vi "eodrecorder_sarah_sam - Timed (2012).vi"() -> ()   [LabVIEW 2013]
uses:
  Dependencies/eodrecorderstates.ctl
  <vilib>/Utility/error.llb/DialogType.ctl
  <vilib>/_DAQmxBase/Internals/DAQmxBase Create Channel (AI-Voltage-Basic).vi
  <vilib>/_DAQmxBase/Internals/DAQmxBase Timing (Sample Clock).vi
  <vilib>/_DAQmxBase/Internals/DAQmxBase Read (Analog 2D DBL NChan NSamp).vi
panel:
  out "String":string
  in  "Length":dbl=0.05
  in  "Device in":tag="Dev1"
  out "Threshold":sgl
  out "?":string="10 E"
  in  "Multiplier":sgl min=-2 max=0
  in  "Modify\nThreshold":dbl(slide) min=0.0 max=9.0 step=1.0 scale=0.0..9.0 scale format="%#_1g"
  in  "?":bool
  out "Number\nof Samples":sgl=10000.0
  in  "Sample Rate":dbl=10000.0
  in  "Channel":tag="Dev1/ai0"
  out "Tab Control":enum32{"Live Data", "Edit Data", "View Data"}(tab)
  in  "Tab Control 2":enum32{"Enter Data", "View Data"}(tab)
  out "Waveforms\nCollected":dbl
  in  "Path":path
  out "Time":string
  out "Date":string
  in  "Specimen No.":string
  in  "Locality Code":string
  in  "Gain":dbl(knob)=10000.0 step=1.0 scale=1.0..50000.0 scale format="%#_6e"
  in  "Coupling":bool
  in  "Recording Temp °C":string
  in  "Comments":string
  in  "Species":string
  in  "StartOver":bool
  in  "Save&Continue":bool
  in  "Save&Finish":bool
  in  "Discard&Continue":bool
  in  "Polarity 2":bool
  in  "Timed":bool
  out "Number of \nWaveforms":dbl caption="Number of Waveforms" format="%#g"
  in  "Wave Number":u16(slide) scale=0.0..1.0
  in  "Polarity":bool
  out "EodText":string[](array[string])
  out "Polarity":i32[](array[numeric])
  out "Npts":i32[](array[numeric])
  out "Srate":i32[](array[numeric])
  out "ADRange":dbl[](array[numeric])
  in  "WaveNumber":i32(slide)=1 min=0 step=1 scale=1.0..3.0 scale format="%#.0f"
  out "Waveform Graph":dbl[][](graph)
  in  "LiveDataMode":bool
  in  "Capture":bool
  in  "Stop":bool
  in  "Open Data":bool
  # "EOD Recorder v. 1.0"
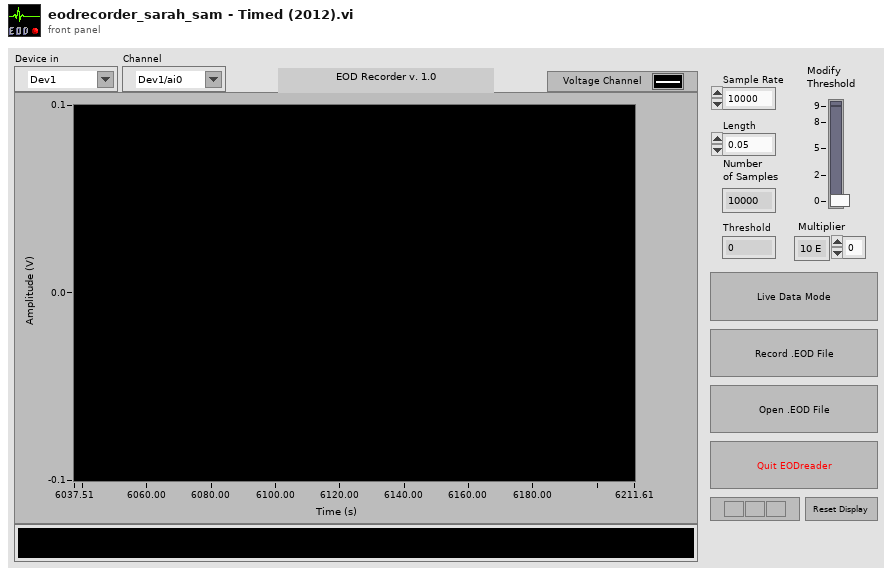
[diagram p1: front panel]
types:
  T1 = cluster{"data":dbl[][], "task ":refnum<k21>, "error ":errorcluster, "Min":dbl, "Max":dbl, "LastGrabbedSrate":dbl, "WaveformData":cluster{"Nchar":i32[], "EodText":string[], "Nbits":i32[], "Nbytes":i32[], "userdata":dbl[][], "Polarity":i32[], "Srate":i32[], "ADRange":dbl[], "Npts":i32[], "Wave":dbl[][]}, "NumberofWavesLoaded":i32, "DescribeWave":cluster{"Specimen 2":string, "Location 2":string, "Species 2":string, "Temp 2":string, "Comments 2":string, "Gain 2":dbl, "Coupling 2":bool, "Date 2":string, "Time 2":string, "Srate 2":dbl, "Polarity 2":bool, "npts":i32}[], "lastgrabbedsamples":i32}
  T2 = typedef "eodrecorderstates.ctl" = enum16{"stop", "initialize", "live data", "capture data", "analyze data", "open data", "display opened data", "write to file"}
  T3 = enum16{"Rising Edge", "Falling Edge", "Above Level", "Below Level", "When Inside Window", "When Outside Window"}
  T4 = enum16{"open", "replace", "create", "open or create", "replace or create", "replace or create with confirmation"}
  T5 = cluster{"Specimen 2":string, "Location 2":string, "Species 2":string, "Temp 2":string, "Comments 2":string, "Gain":dbl, "Coupling":bool, "Date 2":string, "Time 2":string, "Srate":dbl, "Polarity":bool, "npts":i32}
  T6 = typedef "DialogType.ctl" = u16
  T7 = cluster{"Nchar":i32[], "EodText":string[], "Nbits":i32[], "Nbytes":i32[], "userdata":dbl[][], "Polarity":i32[], "Srate":i32[], "ADRange":dbl[], "Npts":i32[], "Wave":dbl[][]}
  T8 = typedef "eventvkey.ctl" = enum16{"ASCII", "Enter", "Return", "Shift", "Ctrl", "Alt", "Cmd", "Opt", "Caps", "NumLock", "Clear", "Break", "Up", "Down", "Left", "Right", "Insert", "Delete", "Home", "End", "PageUp", "PageDown", "Escape", "Help", "Pause", "ScrollLock", "F1", "F2", "F3", "F4", "F5", "F6", "F7", "F8", "F9", "F10", "F11", "F12", "F13", "F14", "F15", "F16", "F17", "F18", "F19", "F20", "F21", "F22", "F23", "F24", "Play", "VolumeUp", "VolumeDown", "Mute", "Two Byte Char"}
  T9 = cluster{"Specimen 2":string, "Location 2":string, "Species 2":string, "Temp 2":string, "Comments 2":string, "Gain 2":dbl, "Coupling 2":bool, "Date 2":string, "Time 2":string, "Srate 2":dbl, "Polarity 2":bool, "npts":i32}[]
  T10 = cluster{"Specimen 2":string, "Location 2":string, "Species 2":string, "Temp 2":string, "Comments 2":string, "Gain 2":dbl, "Coupling 2":bool, "Date 2":string, "Time 2":string, "Srate 2":dbl, "Polarity 2":bool, "npts":i32}
  T11 = cluster{"[0]":bool, "[1]":bool, "[2]":bool, "[3]":bool, "[4]":bool, "[5]":bool, "[6]":bool, "[7]":bool, "[8]":bool}
  T12 = cluster{"Time 2":string, "Date 2":string, "Specimen 2":string, "Location 2":string, "Species 2":string, "Temp 2":string, "Gain 2":dbl, "Coupling 2":bool, "Comments 2":string}
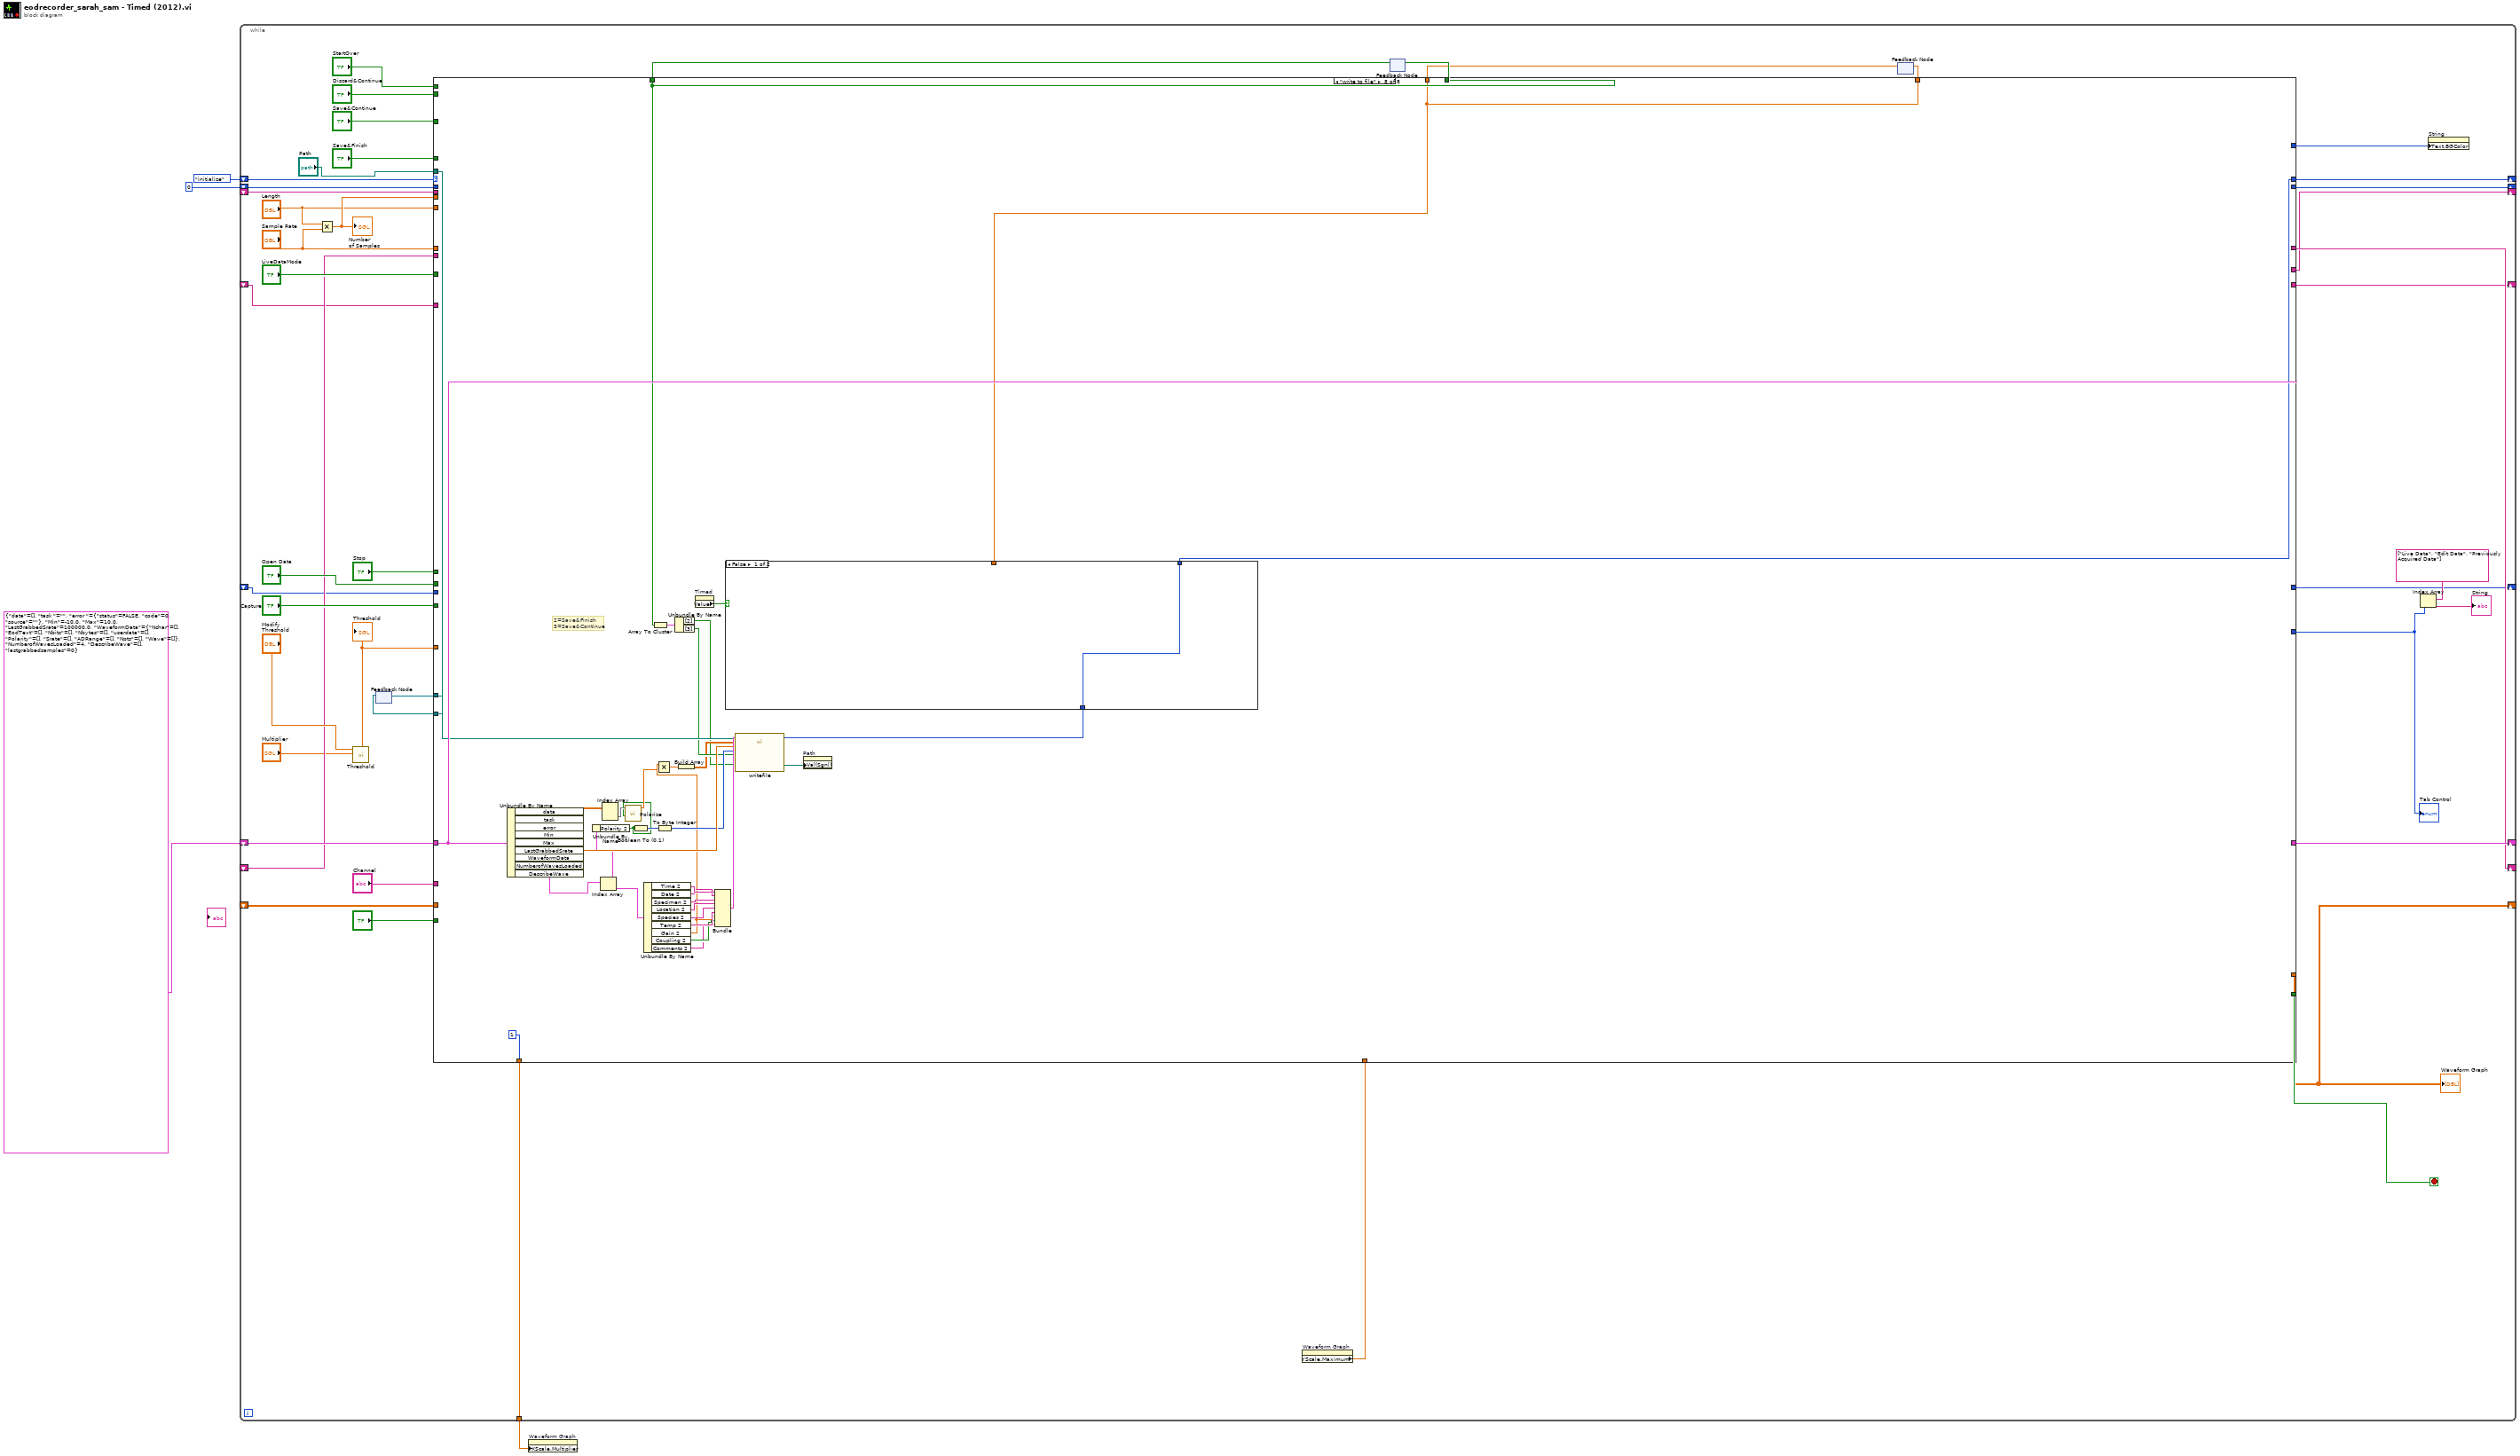
[diagram p0: block diagram]
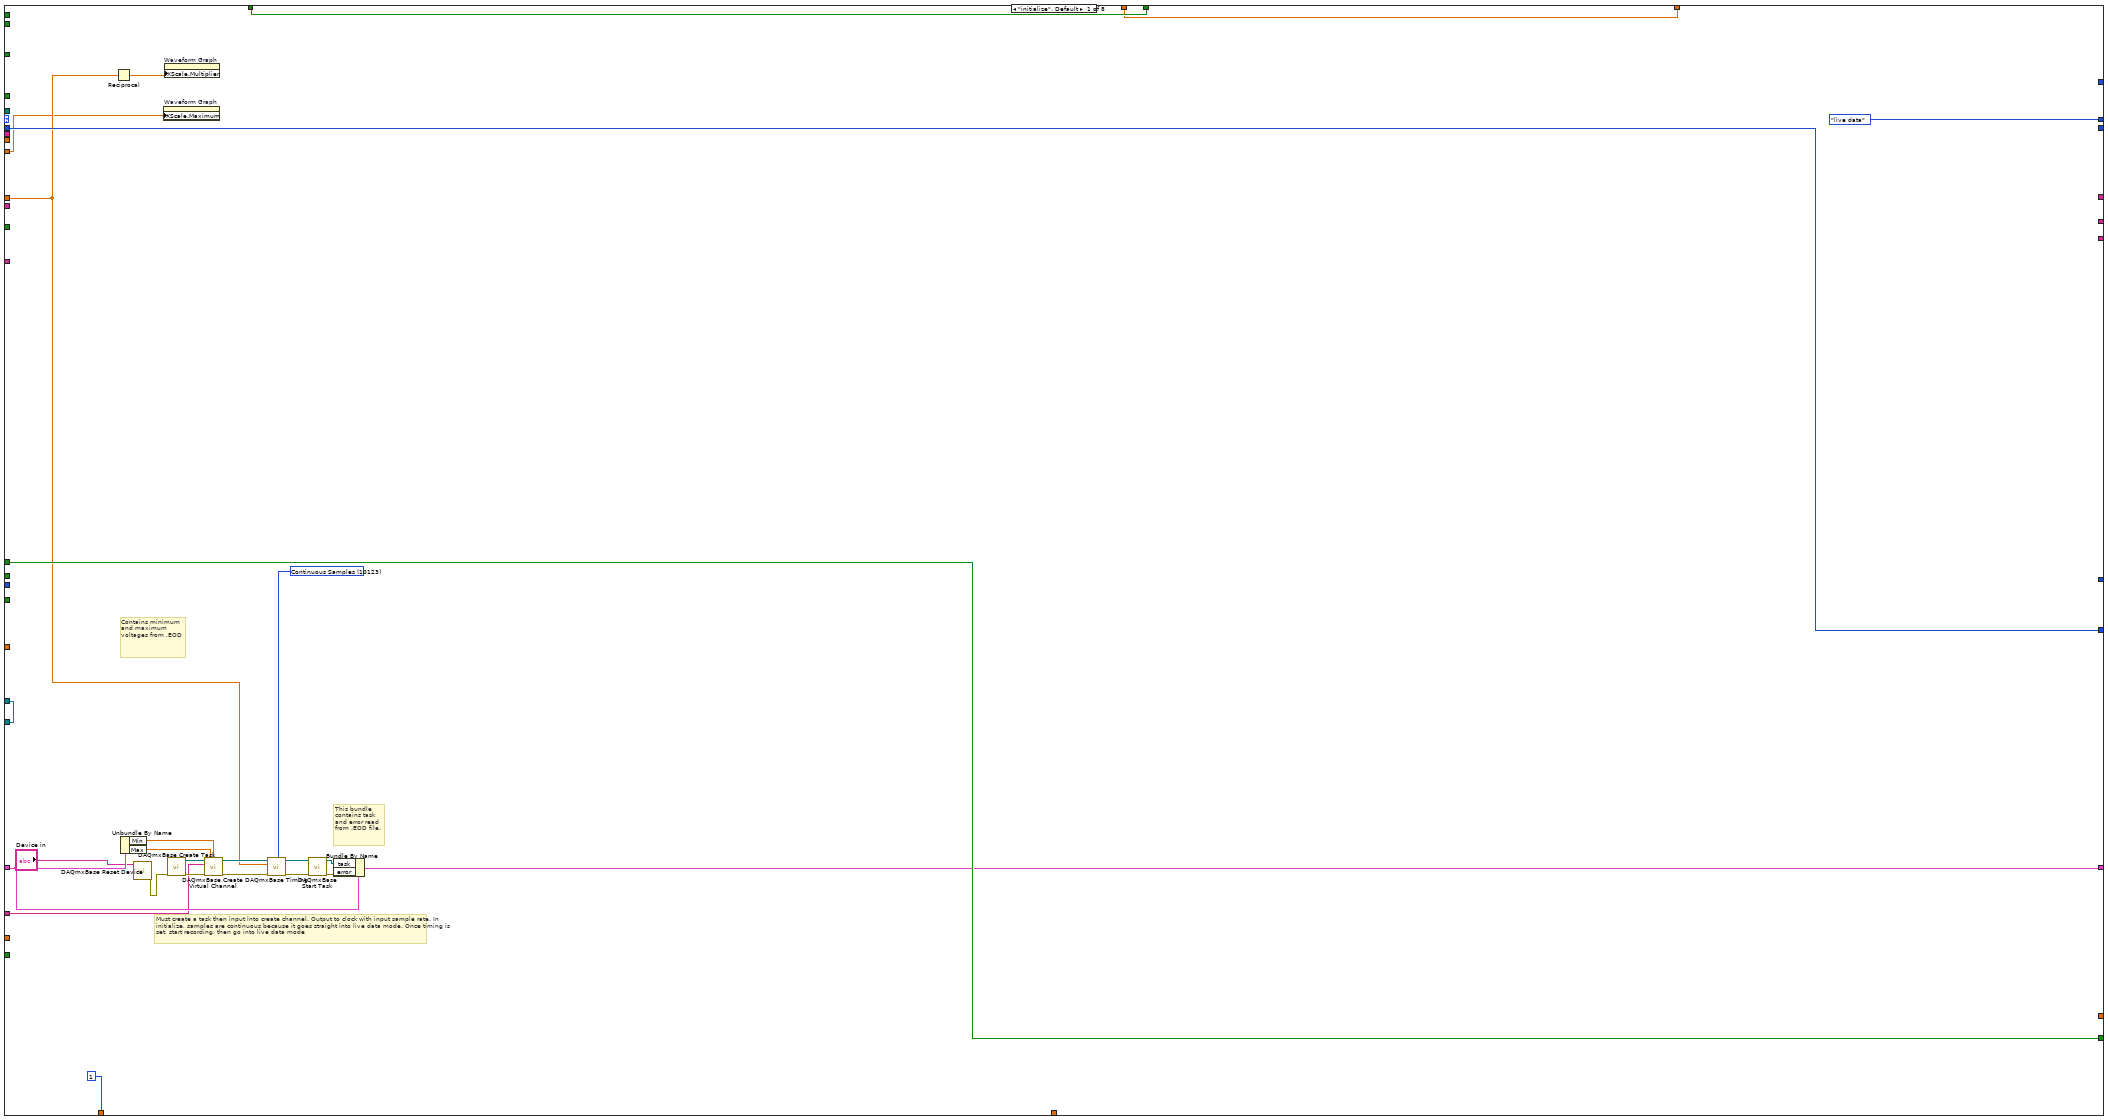
[diagram p2: hidden frame]
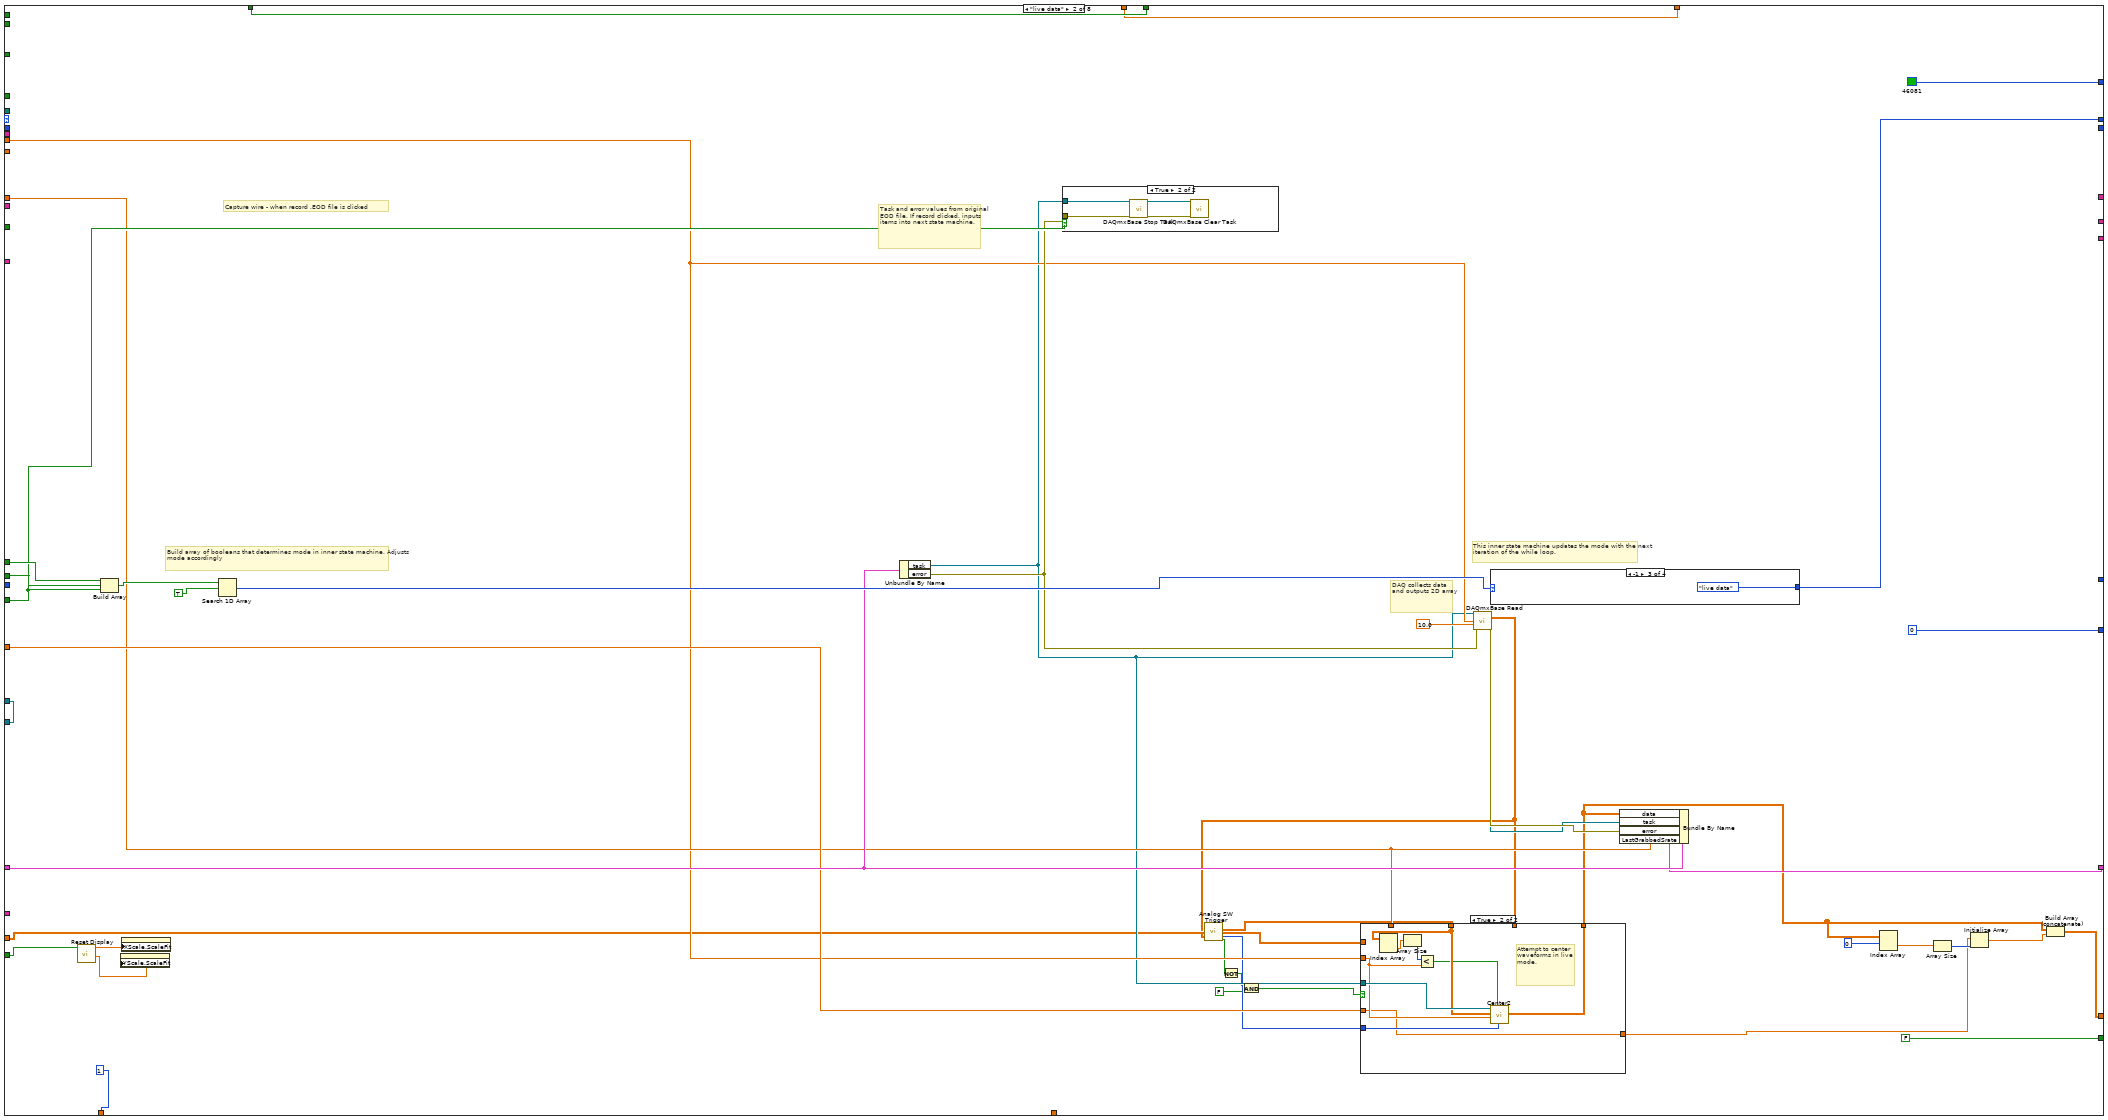
[diagram p3: hidden frame]
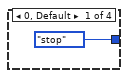
[diagram p6: hidden frame]
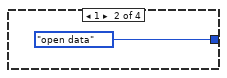
[diagram p7: hidden frame]
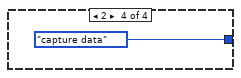
[diagram p8: hidden frame]
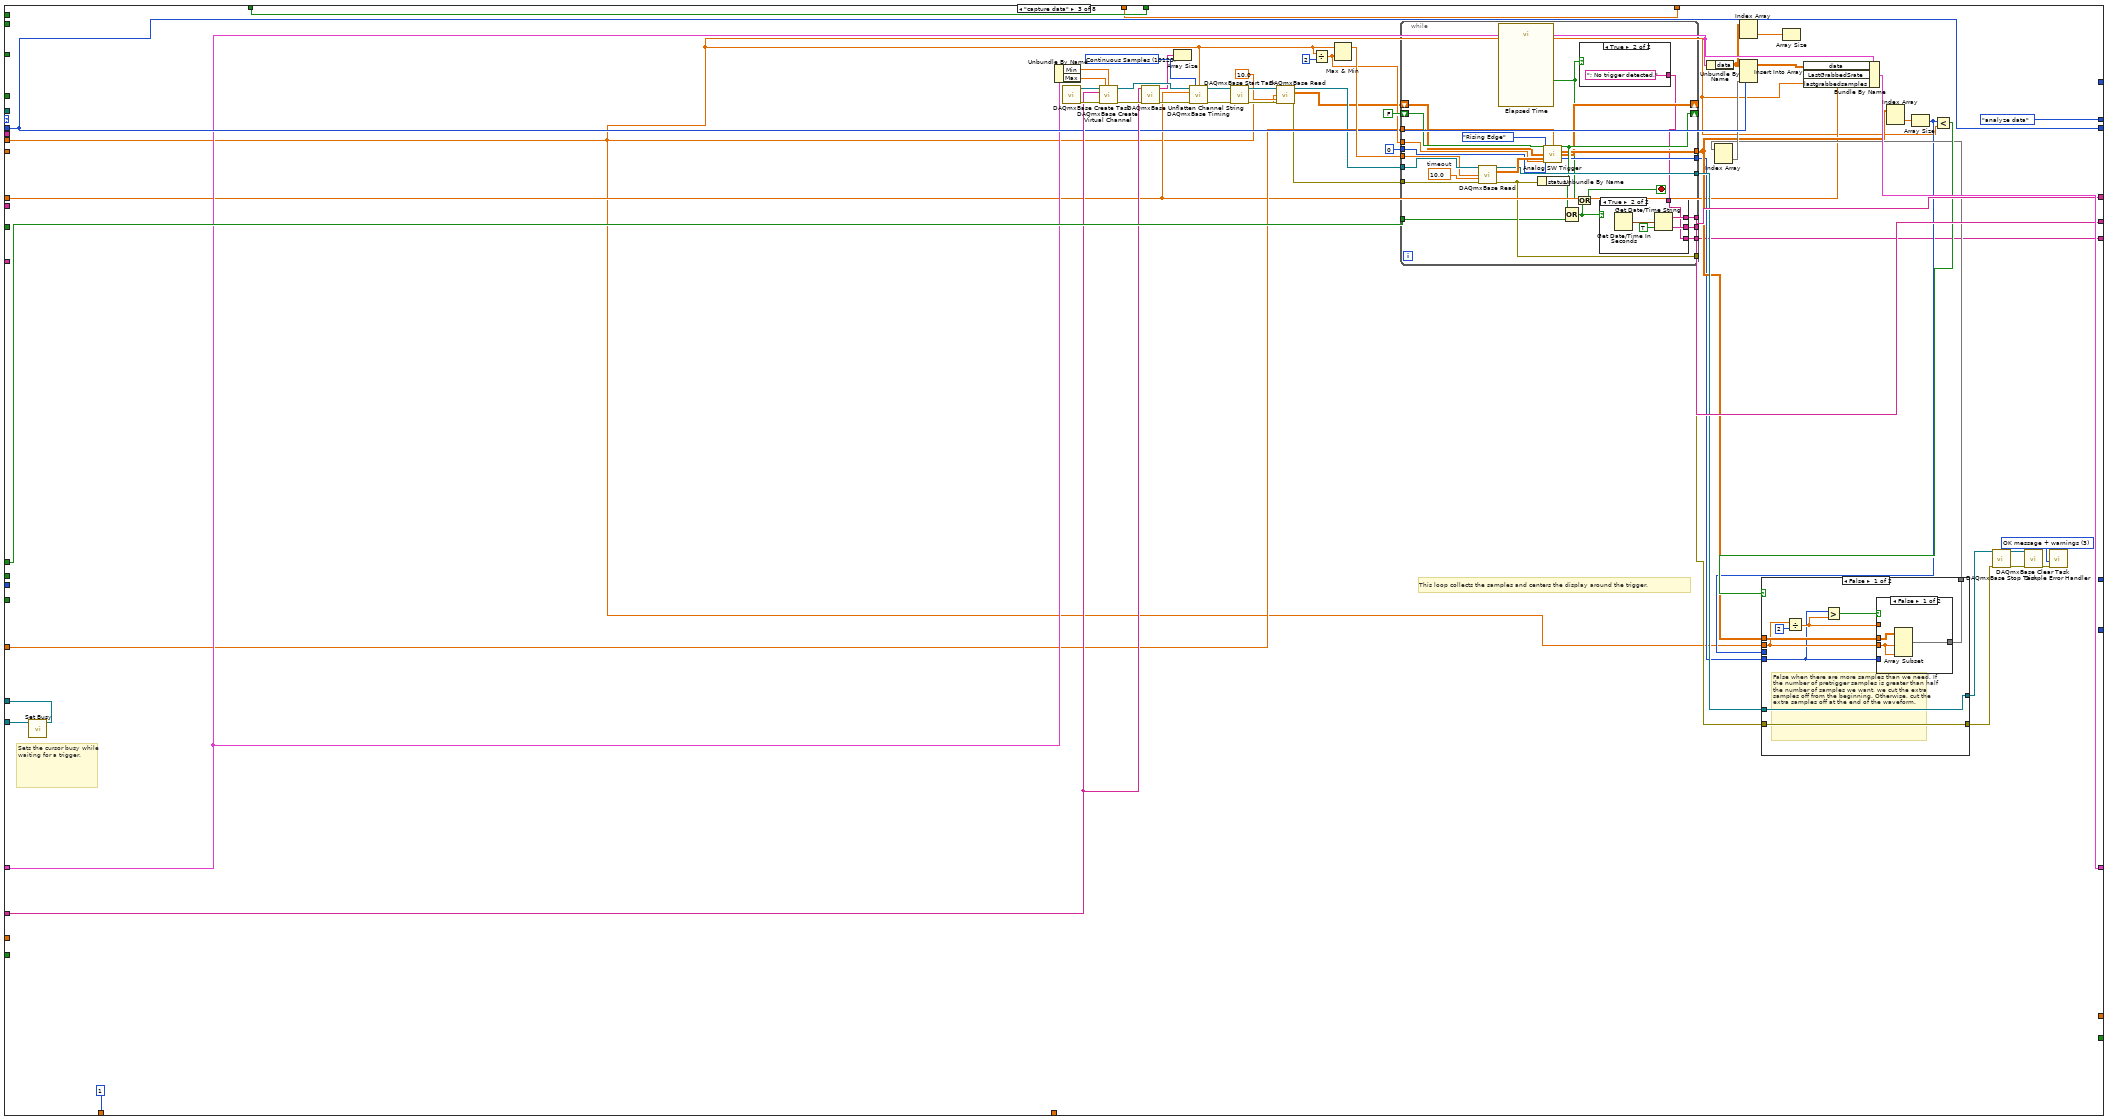
[diagram p9: hidden frame]
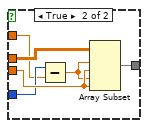
[diagram p10: hidden frame]
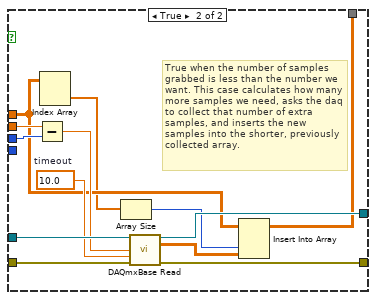
[diagram p11: hidden frame]
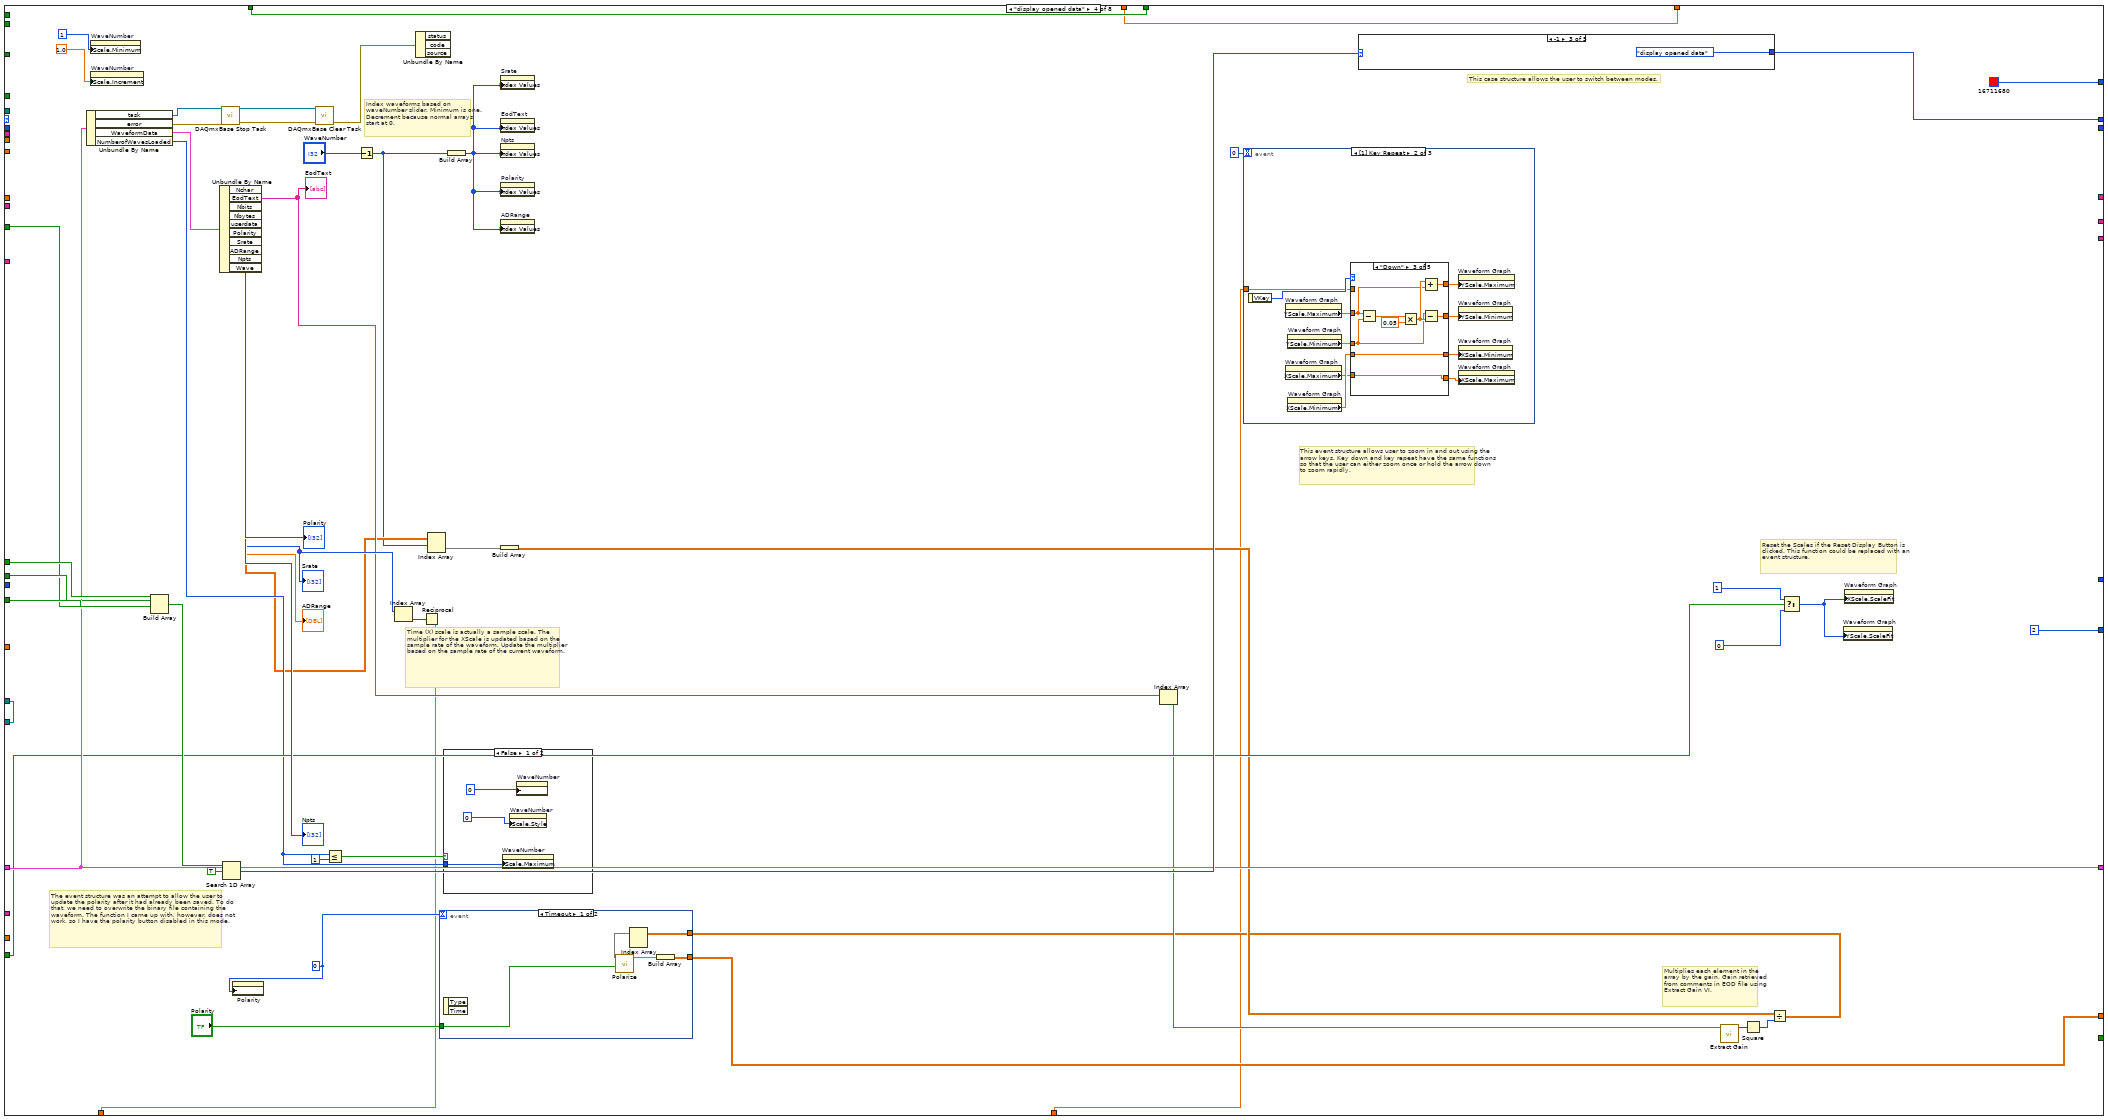
[diagram p14: hidden frame]
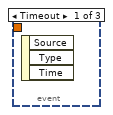
[diagram p15: hidden frame]
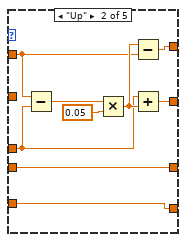
[diagram p17: hidden frame]
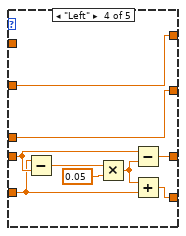
[diagram p18: hidden frame]
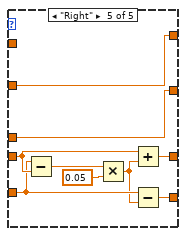
[diagram p19: hidden frame]
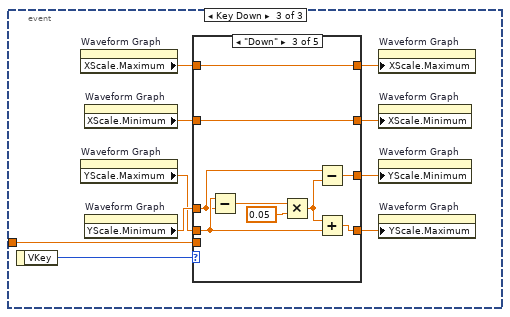
[diagram p20: hidden frame]
diagram:
  n1 = while {
    shift-right: [w49] -> _
    shift-left: eodrecorderstates."initialize" ("Enum") -> [w44]
    shift-right: [w37] -> _
    shift-left: T1 {"data"=[], "task "="", "error "={"status"=FALSE, "code"=0, "source"=""}, "Min"=-10.0, "Max"=10.0, "LastGrabbedSrate"=100000.0, "WaveformData"={"Nchar"=[], "EodText"=[], "Nbits"=[], "Nbytes"=[], "userdata"=[], "Polarity"=[], "Srate"=[], "ADRange"=[], "Npts"=[], "Wave"=[]}, "NumberofWavesLoaded"=4, "DescribeWave"=[], "lastgrabbedsamples"=0} -> [w47]
    shift-right: [w38] -> _
    shift-left: u16 0 -> [w39]
    shift-right: [w35] -> _
    shift-left: _ -> [w26]
    shift-right: [w34] -> _
    shift-left: _ -> [w33]
    shift-right: [w24] -> _
    shift-left: _ -> [w22]
    shift-right: [w12] -> _
    shift-left: _ -> [w11]
    shift-right: [w7] -> _
    shift-left: _ -> [w6]
    tunnel: [w5] -> w1
    stop <- w50 stop-if-true
    n2 = Multiply(x="Length", y="Sample Rate") -> (x*y=w29:dbl)
    "Number\nof Samples" <- w29
    n3 = call "Threshold.vi"("Multiplier"="Multiplier", "Slide"="Modify\nThreshold") -> ("New Threshold"=w27:dbl)  [unwired: 9 in]
    "Threshold" <- w27
    n4 = feedback #1() -> (w15:refnum<k1>)  [unwired: 1 in]
    n5 = property on="Waveform Graph" class="WFGraph (strict)"() -> ("YScale.Maximum"=w8:dbl)  [unwired: 2 in, 2 out]
    n6 = feedback #2() -> (w13:bool[])  [unwired: 1 in]
    n7 = feedback #3() -> (w9:dbl)  [unwired: 1 in]
    n8 = case shown="\"write to file\"" w44 {
      tunnel: [w75 FALSE _ _ _ TRUE w536 _] -> w50
      tunnel: [eodrecorderstates."live data" ("Enum") w118 eodrecorderstates."analyze data" ("Enum") w309 w442 _ w494 w718] -> w49
      tunnel: "Stop" -> [w75 w117 w178 w303 _ _ w536 _]
      tunnel: w47 -> [w63 w113 w169 w286 w440 _ w535 w748]
      tunnel: w29 -> [_ w96 w143 _ _ _ _ _]
      tunnel: "Sample Rate" -> [w56 w99 w152 _ _ _ _ _]
      tunnel: "Open Data" -> [_ w111 _ w305 _ _ _ _]
      tunnel: "Capture" -> [_ w110 _ w306 _ _ _ _]
      tunnel: "LiveDataMode" -> [_ _ _ w302 _ _ _ _]
      tunnel: w27 -> [_ w100 w168 _ _ _ _ _]
      tunnel: [w62 0 _ 2 _ _ 1 _] -> w41
      tunnel: [_ u32 46081 _ u32 16711680 _ _ u32 16773632 _] -> w40
      tunnel: w39 -> [w62 _ w170 _ _ _ w505 _]
      tunnel: [_ _ w170 _ _ _ w503 _] -> w38
      tunnel: [w60 w106 w173 w286 w439 _ w534 w748] -> w37
      tunnel: "Channel" -> [w61 _ w174 _ _ _ _ _]
      tunnel: [_ _ w172 _ _ _ w524 _] -> w35
      tunnel: [_ _ w171 _ _ _ w523 _] -> w34
      tunnel: w26 -> [_ _ _ _ _ _ w524 _]
      tunnel: w33 -> [_ _ _ _ _ _ w523 _]
      tunnel: [_ w80 _ w266 _ _ w513 _] -> w24
      tunnel: "?" -> [_ w103 _ w283 _ _ w511 _]
      tunnel: "Length" -> [w55 _ _ _ _ _ _ _]
      tunnel: w22 -> [_ w92 _ _ _ _ _ _]
      tunnel: "StartOver" -> [_ _ _ _ _ _ _ _]
      tunnel: "Save&Continue" -> [_ _ _ _ _ _ _ _]
      tunnel: "Save&Finish" -> [_ _ _ _ _ _ _ _]
      tunnel: "Discard&Continue" -> [_ _ _ _ _ _ _ _]
      tunnel: "Path" -> [_ _ _ _ _ _ w497 w731]
      tunnel: [1 1 1 w262 1 1 1 1] -> w5
      tunnel: [w53 w97 w149 w277 w436 w484 w509 w728] -> w16
      tunnel: w15 -> [w53 w97 w150 w277 w436 w484 w509 w728]
      tunnel: [w52 w78 w148 w274 w435 w483 w498 w725] -> w14
      tunnel: w13 -> [w52 w78 w148 w274 w435 w483 _ w725]
      tunnel: [_ _ _ _ w433 _ _ _] -> w12
      tunnel: w11 -> [_ _ _ _ _ _ _ _]
      tunnel: [w51 w77 w147 w263 w432 w482 w496 w716] -> w10
      tunnel: w9 -> [w51 w77 w147 w263 w432 w482 w490 w716]
      tunnel: w8 -> [_ _ _ w261 _ _ w489 _]
      tunnel: [_ _ w139 _ _ _ _ _] -> w7
      tunnel: w6 -> [_ _ _ _ _ _ w487 _]
      frame "initialize", Default {
        w70 = 10123 items=["Finite Samples"=10178, "Continuous Samples"=10123] ("sample mode")
        # "Must create a task then input into create channel. Output to clock with input sample rate. In initialize, samples are continuous because it goes straight into live data mode. Once timing is set, start recording, then go into live data mode"
        # "Contains minimum and maximum voltages from .EOD"
        # "This bundle contains task and error read from .EOD file."
        n9 = Reciprocal(x=w56) -> (1/x=w57:dbl)
        n10 = Unbundle By Name(w63) -> ("Min"=w67:dbl, "Max"=w66:dbl)
        n11 = call <vilib>:"DAQmxBase Reset Device.vi"("device in"="Device in") -> ("error out"=w58:errorcluster)  [unwired: 14 in]
        n12 = property on="Waveform Graph" class="WFGraph (strict)"("XScale.Maximum"=w55) -> ()  [unwired: 2 in, 2 out]
        n13 = property on="Waveform Graph" class="WFGraph (strict)"("XScale.Multiplier"=w57) -> ()  [unwired: 2 in, 2 out]
        n14 = call <vilib>:"DAQmxBase Create Task.vi"("error in"=w58) -> ("task out"=w73:refnum<k21>, "error out"=w74:errorcluster)  [unwired: 4 in, 9 out]
        n15 = call-poly <vilib>:"DAQmxBase Create Virtual Channel.vi"("task in"=w73, "maximum value"=w66, "minimum value"=w67, "physical channels"=w61, "error in"=w74) -> ("task out"=w71:refnum<k21>, "error out"=w72:errorcluster)  [unwired: 4 in, 5 out]
        n16 = call-poly <vilib>:"DAQmxBase Timing.vi"("task/channels in"=w71, "sample mode"=w70, "rate"=w56, "error in"=w72) -> ("task out"=w65:refnum<k21>, "error out"=w64:errorcluster)  [unwired: 3 in, 7 out]
        n17 = call <vilib>:"DAQmxBase Start Task.vi"("task/channels in"=w65, "error in"=w64) -> ("task out"=w69:refnum<k21>, "error out"=w68:errorcluster)  [unwired: 12 out]
        n18 = Bundle By Name(cluster=w63, "task"=w69, "error"=w68) -> (w60:T1)
      }
      frame "live data" {
        # "This inner state machine updates the mode with the next iteration of the while loop."
        # "DAQ collects data and outputs 2D array"
        # "Task and error values from original EOD file. If record clicked, inputs items into next state machine."
        # "Capture wire - when record .EOD file is clicked"
        # "Build array of booleans that determines mode in inner state machine. Adjusts mode accordingly"
        n19 = call "Reset Display.vi"("Reset Button"=w103) -> ("YScale Fit"=w101:dbl, "XScale Fit"=w102:dbl)  [unwired: 9 in]
        n20 = Build Array(w117, w111, w110) -> (w116:bool[])
        n21 = property class="WFGraph (strict)"("YScale.ScaleFit"=w101) -> ()  [unwired: 2 in, 2 out]
        n22 = property class="WFGraph (strict)"("XScale.ScaleFit"=w102) -> ()  [unwired: 2 in, 2 out]
        n23 = Search 1D Array(1D array=w116, element=TRUE) -> (index of element=w114:i32)  [unwired: 1 in]
        n24 = Unbundle By Name(w113) -> ("task"=w95:refnum<k21>, "error"=w109:errorcluster)
        n25 = case shown="True" w110 {
          tunnel: w95 -> [_ w134]
          tunnel: w109 -> [_ w133]
          frame False {
          }
          frame True {
            n26 = call <vilib>:"DAQmxBase Stop Task.vi"("task/channels in"=w134, "error in"=w133) -> ("task out"=w132:refnum<k21>, "error out"=w131:errorcluster)  [unwired: 12 in]
            n27 = call <vilib>:"DAQmxBase Clear Task.vi"("task in"=w132, "error in"=w131) -> ()  [unwired: 13 in, 1 out]
          }
        }
        n28 = call-poly <vilib>:"DAQmxBase Read.vi"("task/channels in"=w95, "number of samples per channel"=w96, "timeout"=10.0, "error in"=w109) -> ("task out"=w105:refnum<k21>, "data"=w90:dbl[][], "error out"=w112:errorcluster)  [unwired: 9 out]
        n29 = call "Analog SW Trigger.vi"("Initialized Data Array"=w92, "Input Raw Data"=w90) -> ("Output Data (Scaled)"=w93:dbl[][], "Raw Data Out"=w91:dbl[][], "# Pretrigger Samples"=w94:i32, "Pre-Trigger Error"=w89:bool)  [unwired: 9 in, 1 out]
        n30 = Not(x=w89) -> (.not. x?=w88:bool)
        n31 = And(x=w88, y=FALSE) -> (x .and. y?=w87:bool)
        n32 = case shown="True" w87 {
          tunnel: w100 -> [w120 w122]
          tunnel: w93 -> [_ w127]
          tunnel: w99 -> [_ _]
          tunnel: [w121 w130] -> w81
          tunnel: w96 -> [_ w124]
          tunnel: w95 -> [_ w129]
          tunnel: w94 -> [_ w128]
          tunnel: w91 -> [_ _]
          tunnel: w90 -> [w121 _]
          tunnel: [w120 w122] -> w79
          frame False {
          }
          frame True {
            # "Attempt to center waveforms in live mode."
            n33 = Index Array(array=w127) -> (element=w126:dbl[])  [unwired: 2 in]
            n34 = Array Size(array=w126) -> (size(s)=w125:i32)
            n35 = Less?(x=w125, y=w124) -> (x < y?=w123:bool)
            n36 = call "Center2.vi"("Pretrigger Samples?"=w128, "Not enough Data?"=w123, "Num Samples"=w124, "Data In"=w127, "DAQmx Task In"=w129) -> ("Data Out"=w130:dbl[][])  [unwired: 4 in, 2 out]
          }
        }
        n37 = case shown="-1" w114 {
          tunnel: [eodrecorderstates."stop" ("Enum") eodrecorderstates."open data" ("Enum") eodrecorderstates."live data" ("Enum") eodrecorderstates."capture data" ("Enum")] -> w118
          frame 0, Default {
          }
          frame 1 {
          }
          frame -1 {
          }
          frame 2 {
          }
        }
        n38 = Bundle By Name(cluster=w113, "data"=w81, "task"=w105, "error"=w112, "LastGrabbedSrate"=w99) -> (w106:T1)
        n39 = Index Array(array=w81, index (row)=0) -> (element=w83:dbl[])  [unwired: 1 in]
        n40 = Array Size(array=w83) -> (size(s)=w84:i32)
        n41 = Initialize Array(w79, w84) -> (w82:dbl[])
        n42 = Build Array (concatenate)(w81, w82) -> (w80:dbl[][])
      }
      frame "capture data" {
        w166 = T6 3 items=["no dialog", "OK message", "continue or stop message", "OK message + warnings", "continue/stop + warnings"] ("type of dialog (OK msg:1)")
        w195 = 10123 items=["Finite Samples"=10178, "Continuous Samples"=10123] ("sample mode")
        # "Sets the cursor busy while waiting for a trigger."
        # "This loop collects the samples and centers the display around the trigger."
        n43 = call <vilib>:"Set Busy.vi"("cursor ID"=w150) -> ("previous cursor ID"=w149:refnum<k1>)  [unwired: 9 in, 1 out]
        n44 = Unbundle By Name(w169) -> ("Min"=w192:dbl, "Max"=w191:dbl)
        n45 = call <vilib>:"DAQmxBase Create Task.vi"() -> ("task out"=w194:refnum<k21>, "error out"=w193:errorcluster)  [unwired: 14 in]
        n46 = call-poly <vilib>:"DAQmxBase Create Virtual Channel.vi"("task in"=w194, "maximum value"=w191, "minimum value"=w192, "physical channels"=w174, "error in"=w193) -> ("task out"=w190:refnum<k21>, "error out"=w187:errorcluster)  [unwired: 9 in]
        n47 = call "DAQmxBase Unflatten Channel String.vi"("names in"=w174, "error in"=w187) -> ("names out"=w185:string[], "error out"=w186:errorcluster)  [unwired: 12 in]
        n48 = Array Size(array=w185) -> ()  [unwired: 1 out]
        n49 = call-poly <vilib>:"DAQmxBase Timing.vi"("task/channels in"=w190, "sample mode"=w195, "samples per channel"=w143, "rate"=w152, "error in"=w186) -> ("task out"=w189:refnum<k21>, "error out"=w188:errorcluster)  [unwired: 2 in, 7 out]
        n50 = call <vilib>:"DAQmxBase Start Task.vi"("task/channels in"=w189, "error in"=w188) -> ("task out"=w146:refnum<k21>, "error out"=w145:errorcluster)  [unwired: 12 out]
        n51 = call-poly <vilib>:"DAQmxBase Read.vi"("task/channels in"=w146, "number of samples per channel"=w143, "timeout"=10.0, "error in"=w145) -> ("task out"=w142:refnum<k21>, "data"=w140:dbl[][], "error out"=w141:errorcluster)  [unwired: 9 in]
        n52 = Divide(x=w143, y=2) -> (x/y=w176:dbl)
        n53 = Max & Min(x=w143, y=w176) -> (max(x,y)=w182:dbl)  [unwired: 1 out]
        n54 = while {
          tunnel: [w246] -> w158
          shift-right: [w245] -> _
          shift-left: FALSE ("Trigger Out") -> [w251]
          shift-right: [w232] -> _
          shift-left: w140 -> [w247]
          tunnel: w141 -> [w244]
          tunnel: w142 -> [w243]
          tunnel: w176 -> [w242]
          tunnel: 0 ("Channel Index") -> [w241]
          tunnel: w182 -> [w240]
          tunnel: [w239] -> w155
          tunnel: [w238] -> w160
          tunnel: w178 -> [w237]
          tunnel: w168 -> [w236]
          tunnel: [w234] -> w172
          tunnel: [w233] -> w171
          tunnel: [w231] -> w153
          tunnel: [w229] -> w139
          stop <- w230 stop-if-true
          w252 = 10.0  # timeout
          n55 = call-poly <vilib>:"DAQmxBase Read.vi"("task/channels in"=w243, "number of samples per channel"=w240, "timeout"=w252, "error in"=w244) -> ("task out"=w246:refnum<k21>, "data"=w248:dbl[][], "error out"=w238:errorcluster)  [unwired: 9 in]
          n56 = call "Elapsed Time"() -> ("Time has Elapsed"=w228:bool)  [unwired: 12 in, 7 out]
          n57 = Unbundle By Name(w238) -> ("status"=w250:bool)
          n58 = call "Analog SW Trigger.vi"("Triggered?"=w251, "Condition"=T3."Rising Edge", "Level"=w236, "Initialized Data Array"=w247, "Input Raw Data"=w248, "Pretrigger Samples"=w242, "Index of Condition Channel"=w241) -> ("Trigger Out"=w245:bool, "Output Data (Scaled)"=w239:dbl[][], "Raw Data Out"=w232:dbl[][], "# Pretrigger Samples"=w231:i32)  [unwired: 4 in, 1 out]
          n59 = Compound Arithmetic op=OR(w245, w250, w237) -> (w235:bool)
          n60 = Or(x=w228, y=w235) -> (x .or. y?=w230:bool)
          n61 = case shown="True" w228 {
            tunnel: [_ "; No trigger detected."] -> w227
            frame False {
            }
            frame True {
            }
          }
          n62 = case shown="True" w235 {
            tunnel: [_ w256] -> w234
            tunnel: [_ w255] -> w233
            tunnel: [_ w254] -> w229
            tunnel: w227 -> [_ w254]
            frame False {
            }
            frame True {
              n63 = Get Date/Time In Seconds() -> (seconds since 1Jan1904=w258:timestamp)
              n64 = Get Date/Time String(seconds (now)=w258, want seconds? (F)=TRUE) -> (date string=w256:string, time string=w255:string)  [unwired: 1 in]
            }
          }
        }
        n65 = Unbundle By Name(w169) -> ("data"=w162:dbl[][])
        n66 = Index Array(array=w162) -> (element=w161:dbl[])  [unwired: 2 in]
        n67 = Array Size(array=w161) -> ()  [unwired: 1 out]
        n68 = Index Array(array=w155) -> (element=w163:dbl[])  [unwired: 2 in]
        n69 = Array Size(array=w163) -> (size(s)=w151:i32)
        n70 = Less?(x=w151, y=w143) -> (x < y?=w156:bool)
        n71 = case shown="False" w156 {
          tunnel: w160 -> [w203 w226]
          tunnel: [w203 w225] -> w159
          tunnel: w158 -> [w204 w224]
          tunnel: [w204 w223] -> w157
          tunnel: w143 -> [w198 w219]
          tunnel: w155 -> [w202 w215]
          tunnel: [w201 w218] -> w154
          tunnel: w151 -> [_ w220]
          tunnel: w153 -> [w196 _]
          frame False {
            # "False when there are more samples than we need. If the number of pretrigger samples is greater than half the number of samples we want, we cut the extra samples off from the beginning. Otherwise, cut the extra samples off at the end of the waveform."
            n72 = Divide(x=w198, y=2) -> (x/y=w197:dbl)
            n73 = Greater?(x=w196, y=w197) -> (0:w200:bool)
            n74 = case shown="False" w200 {
              tunnel: w202 -> [w207 w213]
              tunnel: [w206 w212] -> w201
              tunnel: w198 -> [w205 w211]
              tunnel: w197 -> [_ w209]
              tunnel: w196 -> [_ w210]
              frame False {
                n75 = Array Subset(array=w207, length (row)=w205, length (col)=w205) -> (w206:dbl[][])  [unwired: 2 in]
              }
              frame True {
                n76 = Subtract(x=w210, y=w209) -> (x-y=w208:dbl)
                n77 = Array Subset(array=w213, index (row)=w208, length (row)=w211, index (col)=w208, length (col)=w211) -> (w212:dbl[][])
              }
            }
          }
          frame True {
            w222 = 10.0  # timeout
            # "True when the number of samples grabbed is less than the number we want. This case calculates how many more samples we need, asks the daq to collect that number of extra samples, and inserts the new samples into the shorter, previously collected array."
            n78 = Subtract(x=w219, y=w220) -> (x-y=w221:dbl)
            n79 = Index Array(array=w215) -> (element=w214:dbl[])  [unwired: 2 in]
            n80 = Array Size(array=w214) -> (size(s)=w216:i32)
            n81 = call-poly <vilib>:"DAQmxBase Read.vi"("task/channels in"=w224, "number of samples per channel"=w221, "timeout"=w222, "error in"=w226) -> ("task out"=w223:refnum<k21>, "data"=w217:dbl[][], "error out"=w225:errorcluster)  [unwired: 9 in]
            n82 = Insert Into Array(array=w215, index (col)=w216, new element=w217) -> (w218:dbl[][])  [unwired: 1 in]
          }
        }
        n83 = Index Array(array=w154) -> (element=w165:dbl[])  [unwired: 2 in]
        n84 = Insert Into Array(array=w162, index (row)=w170, new element=w165) -> (w164:dbl[][])  [unwired: 1 in]
        n85 = Bundle By Name(cluster=w169, "data"=w164, "LastGrabbedSrate"=w152, "lastgrabbedsamples"=w143) -> (w173:T1)
        n86 = call <vilib>:"DAQmxBase Stop Task.vi"("task/channels in"=w157, "error in"=w159) -> ("task out"=w180:refnum<k21>, "error out"=w179:errorcluster)  [unwired: 12 in]
        n87 = call <vilib>:"DAQmxBase Clear Task.vi"("task in"=w180, "error in"=w179) -> ("error out"=w181:errorcluster)  [unwired: 13 in]
        n88 = call <vilib>:"Simple Error Handler.vi"("type of dialog (OK msg:1)"=w166, "error in (no error)"=w181) -> ()  [unwired: 3 in, 5 out]
      }
      frame "display opened data" {
        w264 = 0
        # "This event structure allows user to zoom in and out using the arrow keys. Key down and key repeat have the same functions so that the user can either zoom once or hold the arrow down to zoom rapidly."
        # "Time (X) scale is actually a sample scale. The multiplier for the XScale is updated based on the sample rate of the waveform. Update the multiplier based on the sample rate of the current waveform."
        # "Index waveforms based on waveNumber slider. Minimum is one. Decrement because normal arrays start at 0."
        # "Reset the Scales if the Reset Display Button is clicked. This function could be replaced with an event structure."
        # "This case structure allows the user to switch between modes."
        # "Multiplies each element in the array by the gain. Gain retrieved from comments in EOD file using Extract Gain VI."
        # "The event structure was an attempt to allow the user to update the polarity after it had already been saved. To do that, we need to overwrite the binary file containing the waveform. The function I came up with, however, does not work, so I have the polarity button disabled in this mode."
        n89 = Unbundle By Name(w286) -> ("task"=w298:refnum<k21>, "error"=w297:errorcluster, "WaveformData"=w296:T7, "NumberofWavesLoaded"=w273:i32)
        n90 = property on="WaveNumber" class="Slide (strict)"("Scale.Minimum"=1) -> ()  [unwired: 2 in, 2 out]
        n91 = property on="WaveNumber" class="Slide (strict)"("Scale.Increment"=1.0 ("Scale.Range:Increment")) -> ()  [unwired: 2 in, 2 out]
        n92 = Build Array(w303, w302, w306, w305) -> (w308:bool[])
        n93 = Unbundle By Name(w296) -> ("EodText"=w272:string[], "Polarity"=→"Polarity":i32[], "Srate"=w282:i32[], "ADRange"=→"ADRange":dbl[], "Npts"=→"Npts":i32[], "Wave"=w269:dbl[][])  [unwired: 4 out]
        "EodText" <- w272
        "Srate" <- w282
        n94 = call <vilib>:"DAQmxBase Stop Task.vi"("task/channels in"=w298, "error in"=w297) -> ("task out"=w299:refnum<k21>, "error out"=w300:errorcluster)  [unwired: 12 in]
        n95 = Search 1D Array(1D array=w308, element=TRUE) -> (index of element=w304:i32)  [unwired: 1 in]
        n96 = property on="Polarity" class="Bool (strict)"("DisabledEnum"=w264) -> ()  [unwired: 2 in, 2 out]
        n97 = call <vilib>:"DAQmxBase Clear Task.vi"("task in"=w299, "error in"=w300) -> ("error out"=w301:errorcluster)  [unwired: 13 in]
        n98 = Less Or Equal?(x=w273, y=1) -> (x <= y?=w276:bool)
        n99 = Decrement(x="WaveNumber") -> (x-1=w268:i32)
        n100 = Index Array(array=w282) -> (element=w279:i32)  [unwired: 1 in]
        n101 = Unbundle By Name(w301) -> ()  [unwired: 3 out]
        n102 = Reciprocal(x=w279) -> (1/x=w262:dbl)
        n103 = Index Array(array=w269, index (row)=w268) -> (element=w290:dbl[])  [unwired: 1 in]
        n104 = case shown="False" w276 {
          tunnel: w273 -> [w422 _]
          frame False {
            n105 = property on="WaveNumber" class="Slide (strict)"("Scale.Maximum"=w422) -> ()  [unwired: 2 in, 2 out]
            n106 = property on="WaveNumber" class="Slide (strict)"("Scale.Style"=0) -> ()  [unwired: 2 in, 2 out]
            n107 = property on="WaveNumber" class="Slide (strict)"("DisabledEnum"=0) -> ()  [unwired: 2 in, 2 out]
          }
          frame True {
            # "Disables slider if there is only one waveform and sets the wavenumber to the first wave."
            n108 = property on="WaveNumber" class="Slide (strict)"("Scale.Maximum"=2) -> ()  [unwired: 2 in, 2 out]
            n109 = property on="WaveNumber" class="Slide (strict)"("Val(Sgnl)"=1) -> ()  [unwired: 2 in, 2 out]
            n110 = property on="WaveNumber" class="Slide (strict)"("Scale.Style"=5) -> ()  [unwired: 2 in, 2 out]
            n111 = property on="WaveNumber" class="Slide (strict)"("DisabledEnum"=2) -> ()  [unwired: 2 in, 2 out]
          }
        }
        n112 = Build Array(w268) -> (w292:i32[])
        n113 = property on="Srate" class="Arr (strict)"("Index Values"=w292) -> ()  [unwired: 2 in, 2 out]
        n114 = property on="EodText" class="Arr (strict)"("Index Values"=w292) -> ()  [unwired: 2 in, 2 out]
        n115 = property on="Npts" class="Arr (strict)"("Index Values"=w292) -> ()  [unwired: 2 in, 2 out]
        n116 = property on="Polarity" class="Arr (strict)"("Index Values"=w292) -> ()  [unwired: 2 in, 2 out]
        n117 = property on="ADRange" class="Arr (strict)"("Index Values"=w292) -> ()  [unwired: 2 in, 2 out]
        n118 = Build Array(w290) -> (w281:dbl[][])
        n119 = Index Array(array=w272) -> (element=w270:string)  [unwired: 1 in]
        n120 = event shown="[1] Key Repeat" {
          selector: _ -> [_ _ _]
          dyn-events: _ -> [_ _ _]
          timeout: 0 -> [_ _ _]
          tunnel: w261 -> [_ w310 w360]
          event Timeout {
            n121 = event-data() -> ()  [unwired: 1 in, 3 out]
          }
          event Key Repeat {
            n122 = event-data() -> ("VKey"=w319:T8)  [unwired: 1 in]
            n123 = property on="Waveform Graph" class="WFGraph (strict)"() -> ("YScale.Maximum"=w311:dbl)  [unwired: 2 in, 2 out]
            n124 = property on="Waveform Graph" class="WFGraph (strict)"() -> ("XScale.Maximum"=w313:dbl)  [unwired: 2 in, 2 out]
            n125 = property on="Waveform Graph" class="WFGraph (strict)"() -> ("YScale.Minimum"=w312:dbl)  [unwired: 2 in, 2 out]
            n126 = property on="Waveform Graph" class="WFGraph (strict)"() -> ("XScale.Minimum"=w314:dbl)  [unwired: 2 in, 2 out]
            n127 = case shown="\"Down\"" w319 {
              tunnel: w314 -> [w323 w332 w341 w348 w357]
              tunnel: [w323 w332 w341 w345 w354] -> w317
              tunnel: w313 -> [w322 w331 w340 w342 w352]
              tunnel: [w322 w331 w340 w344 w353] -> w318
              tunnel: w312 -> [w321 w324 w333 w350 w359]
              tunnel: w311 -> [w320 _ w336 w349 w358]
              tunnel: [w321 w326 w335 w350 w359] -> w316
              tunnel: [w320 w325 w334 w349 w358] -> w315
              tunnel: w310 -> [_ w327 _ _ _]
              frame Default {
              }
              frame "Up" {
                n128 = Subtract(x=w327, y=w324) -> (x-y=w329:dbl)
                n129 = Multiply(x=w329, y=0.05) -> (x*y=w328:dbl)
                n130 = Subtract(x=w328, y=w327) -> (x-y=w325:dbl)
                n131 = Add(x=w324, y=w328) -> (x+y=w326:dbl)
              }
              frame "Down" {
                n132 = Subtract(x=w336, y=w333) -> (x-y=w338:dbl)
                n133 = Multiply(x=w338, y=0.05) -> (x*y=w337:dbl)
                n134 = Add(x=w337, y=w336) -> (x+y=w334:dbl)
                n135 = Subtract(x=w333, y=w337) -> (x-y=w335:dbl)
              }
              frame "Left" {
                n136 = Subtract(x=w342, y=w348) -> (x-y=w346:dbl)
                n137 = Multiply(x=w346, y=0.05) -> (x*y=w343:dbl)
                n138 = Subtract(x=w348, y=w343) -> (x-y=w345:dbl)
                n139 = Add(x=w343, y=w342) -> (x+y=w344:dbl)
              }
              frame "Right" {
                n140 = Subtract(x=w352, y=w357) -> (x-y=w355:dbl)
                n141 = Multiply(x=w355, y=0.05) -> (x*y=w351:dbl)
                n142 = Add(x=w357, y=w351) -> (x+y=w354:dbl)
                n143 = Subtract(x=w352, y=w351) -> (x-y=w353:dbl)
              }
            }
            n144 = property on="Waveform Graph" class="WFGraph (strict)"("YScale.Maximum"=w315) -> ()  [unwired: 2 in, 2 out]
            n145 = property on="Waveform Graph" class="WFGraph (strict)"("YScale.Minimum"=w316) -> ()  [unwired: 2 in, 2 out]
            n146 = property on="Waveform Graph" class="WFGraph (strict)"("XScale.Minimum"=w317) -> ()  [unwired: 2 in, 2 out]
            n147 = property on="Waveform Graph" class="WFGraph (strict)"("XScale.Maximum"=w318) -> ()  [unwired: 2 in, 2 out]
          }
          event Key Down {
            n148 = event-data() -> ("VKey"=w369:T8)  [unwired: 1 in]
            n149 = property on="Waveform Graph" class="WFGraph (strict)"() -> ("XScale.Maximum"=w363:dbl)  [unwired: 2 in, 2 out]
            n150 = property on="Waveform Graph" class="WFGraph (strict)"() -> ("YScale.Maximum"=w361:dbl)  [unwired: 2 in, 2 out]
            n151 = property on="Waveform Graph" class="WFGraph (strict)"() -> ("XScale.Minimum"=w364:dbl)  [unwired: 2 in, 2 out]
            n152 = property on="Waveform Graph" class="WFGraph (strict)"() -> ("YScale.Minimum"=w362:dbl)  [unwired: 2 in, 2 out]
            n153 = case shown="\"Down\"" w369 {
              tunnel: w364 -> [w373 w382 w391 w398 w407]
              tunnel: [w373 w382 w391 w395 w404] -> w367
              tunnel: w363 -> [w372 w381 w390 w392 w402]
              tunnel: [w372 w381 w390 w394 w403] -> w368
              tunnel: w362 -> [w371 w374 w383 w400 w409]
              tunnel: w361 -> [w370 _ w386 w399 w408]
              tunnel: [w371 w376 w385 w400 w409] -> w366
              tunnel: [w370 w375 w384 w399 w408] -> w365
              tunnel: w360 -> [_ w377 _ _ _]
              frame Default {
              }
              frame "Up" {
                n154 = Subtract(x=w377, y=w374) -> (x-y=w379:dbl)
                n155 = Multiply(x=w379, y=0.05) -> (x*y=w378:dbl)
                n156 = Add(x=w374, y=w378) -> (x+y=w376:dbl)
                n157 = Subtract(x=w378, y=w377) -> (x-y=w375:dbl)
              }
              frame "Down" {
                n158 = Subtract(x=w386, y=w383) -> (x-y=w388:dbl)
                n159 = Multiply(x=w388, y=0.05) -> (x*y=w387:dbl)
                n160 = Subtract(x=w383, y=w387) -> (x-y=w385:dbl)
                n161 = Add(x=w387, y=w386) -> (x+y=w384:dbl)
              }
              frame "Left" {
                n162 = Subtract(x=w392, y=w398) -> (x-y=w396:dbl)
                n163 = Multiply(x=w396, y=0.05) -> (x*y=w393:dbl)
                n164 = Add(x=w393, y=w392) -> (x+y=w394:dbl)
                n165 = Subtract(x=w398, y=w393) -> (x-y=w395:dbl)
              }
              frame "Right" {
                n166 = Subtract(x=w402, y=w407) -> (x-y=w405:dbl)
                n167 = Multiply(x=w405, y=0.05) -> (x*y=w401:dbl)
                n168 = Subtract(x=w402, y=w401) -> (x-y=w403:dbl)
                n169 = Add(x=w407, y=w401) -> (x+y=w404:dbl)
              }
            }
            n170 = property on="Waveform Graph" class="WFGraph (strict)"("XScale.Maximum"=w368) -> ()  [unwired: 2 in, 2 out]
            n171 = property on="Waveform Graph" class="WFGraph (strict)"("XScale.Minimum"=w367) -> ()  [unwired: 2 in, 2 out]
            n172 = property on="Waveform Graph" class="WFGraph (strict)"("YScale.Minimum"=w366) -> ()  [unwired: 2 in, 2 out]
            n173 = property on="Waveform Graph" class="WFGraph (strict)"("YScale.Maximum"=w365) -> ()  [unwired: 2 in, 2 out]
          }
        }
        n174 = case shown="-1" w304 {
          tunnel: [eodrecorderstates."stop" ("Enum") eodrecorderstates."initialize" ("Enum") eodrecorderstates."display opened data" ("Enum") eodrecorderstates."open data" ("Enum") eodrecorderstates."capture data" ("Enum")] -> w309
          frame 0, Default {
          }
          frame 1 {
          }
          frame -1 {
          }
          frame 3 {
          }
          frame 2 {
          }
        }
        n175 = call "Extract Gain.vi"("EOD Text"=w270) -> ("Gain"=w271:i32)  [unwired: 10 in]
        n176 = Square(x=w271) -> (x^2=w259:i32)
        n177 = Divide(x=w281, y=w259) -> (x/y=w267:dbl[][])
        n178 = event shown="[0] Timeout" {
          selector: _ -> [_ _]
          dyn-events: _ -> [_ _]
          timeout: w264 -> [_ _]
          tunnel: w267 -> [w414 w419]
          tunnel: [w411 w415] -> w266
          tunnel: "Polarity" -> [w410 _]
          event Timeout {
            n179 = event-data() -> ()  [unwired: 1 in, 2 out]
            n180 = Index Array(array=w414) -> (element=w413:dbl[])  [unwired: 2 in]
            n181 = call "Polarize.vi"("Polarity"=w410, "Wave array"=w413) -> ("Inverse Wave Array"=w412:dbl[])  [unwired: 9 in]
            n182 = Build Array(w412) -> (w411:dbl[][])
          }
          event "Polarity": Value Change {
            n183 = event-data() -> ("NewVal"=w417:bool)  [unwired: 1 in, 4 out]
            n184 = Index Array(array=w419) -> (element=w418:dbl[])  [unwired: 2 in]
            n185 = call "Polarize.vi"("Polarity"=w417, "Wave array"=w418) -> ("Inverse Wave Array"=w416:dbl[])  [unwired: 9 in]
            n186 = Build Array(w416) -> (w415:dbl[][])
          }
        }
        n187 = Select(t=1, s=w283, f=0) -> (s? t:f=w280:i32)
        n188 = property on="Waveform Graph" class="WFGraph (strict)"("YScale.ScaleFit"=w280) -> ()  [unwired: 2 in, 2 out]
        n189 = property on="Waveform Graph" class="WFGraph (strict)"("XScale.ScaleFit"=w280) -> ()  [unwired: 2 in, 2 out]
      }
      frame "open data" {
        n190 = File Dialog() -> (0:w441:errorcluster, 1:w437:bool, 3:w434:path)  [unwired: 7 in, 1 out]
        n191 = case shown="False" w437 {
          tunnel: [eodrecorderstates."display opened data" ("Enum") eodrecorderstates."initialize" ("Enum")] -> w442
          tunnel: w441 -> [w474 _]
          tunnel: w440 -> [w447 w481]
          tunnel: [w445 w481] -> w439
          tunnel: w434 -> [w444 _]
          tunnel: [w443 w478] -> w433
          frame False {
            # "Get file size"
            n192 = Open/Create/Replace File(file path (use dialog)=w444, error in=w474, operation (0:open)=T4."open", access (0:read/write)=enum16{"read/write", "read-only", "write-only"}."read-only") -> (refnum out=w463:refnum<file>, error out=w456:errorcluster)  [unwired: 2 in, 1 out]
            n193 = Get File Size(file=w463) -> (refnum out=w462:refnum<file>, size (in bytes)=w461:i64)  [unwired: 1 in, 1 out]
            n194 = Unbundle By Name(w447) -> ("WaveformData"=w473:T7)
            n195 = call "openeod.vi"("Byte Stream File in"=w462, "size (in bytes)"=w461, "error in (no error)"=w456) -> ("Wave"=w446:i16[][], "Wave Offset"=w443:i32[], "nchar"=w472:u8[], "polarity"=w468:i8[], "nWavepoints"=w464:u32[], "userdata"=w467:sgl[][], "Numeric"=w459:i32, "nbytes"=w469:i8[], "Byte Stream File out"=w458:refnum<file>, "ADrange"=w465:sgl[], "eodtext"=w471:string[], "srate"=w466:u32[], "nbits"=w470:i8[], "error out"=w457:errorcluster)  [unwired: 3 in]
            n196 = Bundle By Name(cluster=w473, "Nchar"=w472, "EodText"=w471, "Nbits"=w470, "Nbytes"=w469, "userdata"=w467, "Polarity"=w468, "Srate"=w466, "ADRange"=w465, "Npts"=w464, "Wave"=w446) -> (w460:T7)
            n197 = Close File(refnum=w458, error in=w457) -> (error out=w448:errorcluster)  [unwired: 1 out]
            n198 = Bundle By Name(cluster=w447, "WaveformData"=w460, "NumberofWavesLoaded"=w459) -> (w445:T1)
            n199 = Unbundle By Name(w448) -> ("code"=w455:i32)
            n200 = Equal?(x=w455, y=4) -> (x = y?=w453:bool)
            n201 = Select(t=FALSE, s=w453, f=TRUE) -> (s? t:f=w450:bool)
            n202 = Bundle By Name(cluster=w448, "status"=w450) -> (w449:errorcluster)
            n203 = call <vilib>:"Simple Error Handler.vi"("error in (no error)"=w449) -> ()  [unwired: 4 in, 5 out]
          }
          frame True {
            n204 = Build Array(0) -> (w478:i32[])
          }
        }
      }
      frame "stop" {
      }
      frame "analyze data" {
        # "Events structure deciding what to do with the collected waveform. Ctrl+S for Save&Finish must be toggled manually because alphabetical keystrokes are not an option to be toggled on the front panel."
        # "0=Start Over\n1=Discard& Cont\n2=Save&Finish\n3=Save&Continue"
        n205 = call <vilib>:"Unset Busy.vi"() -> ()  [unwired: 11 in, 1 out]
        n206 = property on="Wave Number" class="Slide (strict)"("Scale.Maximum"=w505, "Scale.Minimum"=0.0 ("Scale.Range:Minimum")) -> ()  [unwired: 2 in, 2 out]
        n207 = call "Reset Display.vi"("Reset Button"=w511) -> ("YScale Fit"=w517:dbl, "XScale Fit"=w518:dbl)  [unwired: 9 in]
        n208 = Unbundle By Name(w535) -> ("data"=w522:dbl[][], "LastGrabbedSrate"=w512:dbl, "DescribeWave"=w533:T9, "lastgrabbedsamples"=w519:i32)
        n209 = Build Array("Wave Number") -> ()  [unwired: 1 out]
        n210 = property on="Waveform Graph" class="WFGraph (strict)"("XScale.ScaleFit"=w518) -> ()  [unwired: 2 in, 2 out]
        n211 = property class="WFGraph (strict)"("YScale.ScaleFit"=w517) -> ()  [unwired: 2 in, 2 out]
        n212 = Index Array(array=w522, index (row)="Wave Number") -> (element=w514:dbl[])  [unwired: 1 in]
        n213 = Concatenate Strings("Comments", w487) -> (w488:string)
        n214 = Bundle By Name(cluster=T5 {"Specimen 2"="", "Location 2"="", "Species 2"="", "Temp 2"="", "Comments 2"="", "Gain"=50.0, "Coupling"=TRUE, "Date 2"="", "Time 2"="", "Srate"=0.0, "Polarity"=FALSE, "npts"=0} ("WaveformDescribe 2"), "Specimen 2"="Specimen No.", "Location 2"="Locality Code", "Species 2"="Species", "Temp 2"="Recording Temp °C", "Comments 2"=w488, "Gain"="Gain", "Coupling"="Coupling", "Date 2"=w524, "Time 2"=w523, "Srate"=w512, "Polarity"="Polarity 2", "npts"=w519) -> (w525:T5)
        n215 = Insert Into Array(array=w533, index=w505, new element=w525) -> (w506:T9)
        n216 = call "Polarize.vi"("Polarity"="Polarity 2", "Wave array"=w514) -> ("Inverse Wave Array"=w515:dbl[])  [unwired: 9 in]
        n217 = Build Array(w515) -> (w513:dbl[][])
        n218 = property on="Timed" class="Bool (strict)"() -> ("Value"=w495:bool)  [unwired: 2 in, 2 out]
        n219 = case shown="False" w495 {
          selector: w495 -> [w539 _]
          tunnel: [w539 w542] -> w491
          tunnel: [_ w541] -> w492
          frame False {
          }
          frame True {
            n220 = property on="Waveforms\nCollected" class="DigNum (strict)"() -> ("Value"=w540:dbl)  [unwired: 2 in, 2 out]
            n221 = property on="Number of \nWaveforms" class="DigNum (strict)"() -> ("Value"=w543:dbl)  [unwired: 2 in, 2 out]
            n222 = Less Or Equal?(x=w540, y=w543) -> (x <= y?=w542:bool)
            n223 = case shown="False" w542 {
              tunnel: [eodrecorderstates."stop" ("Enum") eodrecorderstates."write to file" ("Enum")] -> w541
              frame False {
              }
              frame True {
              }
            }
          }
        }
        n224 = event shown="[6] Key Repeat" {
          selector: _ -> [_ _ _ _ _ _ _ _ _]
          dyn-events: _ -> [_ _ _ _ _ _ _ _ _]
          timeout: 0 -> [_ _ _ _ _ _ _ _ _]
          tunnel: w497 -> [_ _ _ w564 _ _ _ _ w705]
          tunnel: w506 -> [w547 w550 w557 w559 w577 w589 w655 w696 _]
          tunnel: w505 -> [_ _ w556 _ w576 _ _ _ _]
          tunnel: [w547 w550 w557 w559 w577 w589 w655 w696 w704] -> w504
          tunnel: [eodrecorderstates."analyze data" ("Enum") _ eodrecorderstates."write to file" ("Enum") w563 eodrecorderstates."write to file" ("Enum") w590 eodrecorderstates."analyze data" ("Enum") eodrecorderstates."capture data" ("Enum") eodrecorderstates."initialize" ("Enum")] -> w493
          tunnel: [_ _ w556 _ w576 _ _ _ 0] -> w503
          tunnel: [_ _ _ _ _ _ _ _ w701] -> w502
          tunnel: [_ _ _ _ _ _ _ w698 _] -> w501
          tunnel: [_ _ w554 _ _ w591 _ _ _] -> w500
          tunnel: [w546 _ _ w562 w574 _ _ _ _] -> w499
          tunnel: [w548 w551 w553 w560 w573 w588 w654 w697 w700] -> w496
          tunnel: w491 -> [w546 _ _ w561 _ _ _ _ _]
          tunnel: w490 -> [w548 w551 w553 _ w573 w588 w654 w697 w700]
          tunnel: w489 -> [_ _ _ _ _ w579 w644 _ _]
          event Timeout {
            # "Remains in analyze mode on the current waveform if none of the buttons are clicked."
            n225 = event-data() -> ()  [unwired: 1 in, 2 out]
          }
          event Panel Close? {
            n226 = event-data() -> ()  [unwired: 1 in, 3 out]
            n227 = event-data("Discard?"=TRUE) -> ()  [unwired: 1 in, 1 out]
          }
          event "Save&Finish": Value Change {
            # "Write to file and update value in button array. Specific instructions in write to file mode."
            n228 = event-data() -> ("NewVal"=w554:bool)  [unwired: 1 in, 4 out]
          }
          event "Timed": Value Change {
            n229 = event-data() -> ("NewVal"=w558:bool)  [unwired: 1 in, 4 out]
            n230 = Or(x=w561, y=w558) -> (x .or. y?=w562:bool)
            n231 = case shown="True" w558 {
              tunnel: w564 -> [_ w572]
              tunnel: [_ eodrecorderstates."write to file" ("Enum")] -> w563
              tunnel: [_ w567] -> w560
              frame False {
              }
              frame True {
                n232 = call "File Dialog"("start path"=w572, "default name"="New Timed") -> ("selected path"=w571:path)  [unwired: 10 in, 3 out]
                n233 = property on="Path" class="Path"("Val(Sgnl)"=w571) -> ()  [unwired: 2 in, 2 out]
                n234 = call "Prompt User for Input"() -> ("Number of Waveforms"=→"Number of \nWaveforms":dbl, "Time Between Waveforms (min)"=w569:dbl)  [unwired: 16 in, 2 out]
                n235 = Multiply(x=w569, y=60.0) -> (x*y=w567:dbl)
              }
            }
          }
          event "Save&Continue": Value Change {
            # "Specific instructions in write to file mode."
            n236 = event-data() -> ("NewVal"=w574:bool)  [unwired: 1 in, 4 out]
          }
          event Key Down {
            # "ScanCode for 's' is 31. So when platmod for Ctrl is activated and S is pressed,  sends VI to write to file mode and updates the value in the button array as if save&finish had been clicked."
            n237 = event-data() -> ("ScanCode"=w593:i16, "PlatMods.Ctrl"=w592:bool, "VKey"=w578:T8)  [unwired: 1 in]
            n238 = property on="Waveform Graph" class="WFGraph (strict)"() -> ("YScale.Maximum"=w580:dbl)  [unwired: 2 in, 2 out]
            n239 = property on="Waveform Graph" class="WFGraph (strict)"() -> ("XScale.Maximum"=w582:dbl)  [unwired: 2 in, 2 out]
            n240 = property on="Waveform Graph" class="WFGraph (strict)"() -> ("YScale.Minimum"=w581:dbl)  [unwired: 2 in, 2 out]
            n241 = property on="Waveform Graph" class="WFGraph (strict)"() -> ("XScale.Minimum"=w583:dbl)  [unwired: 2 in, 2 out]
            n242 = case shown="31" w593 {
              tunnel: [FALSE w636] -> w591
              tunnel: w592 -> [_ w637]
              tunnel: [eodrecorderstates."analyze data" ("Enum") w638] -> w590
              frame 0, Default {
              }
              frame 31 {
                n243 = case shown="True" w637 {
                  selector: w637 -> [w640 w641]
                  tunnel: [eodrecorderstates."analyze data" ("Enum") eodrecorderstates."write to file" ("Enum")] -> w638
                  tunnel: [w640 w641] -> w636
                  frame False {
                  }
                  frame True {
                  }
                }
              }
            }
            n244 = case shown="\"Down\"" w578 {
              tunnel: w583 -> [w597 w606 w615 w622 w631]
              tunnel: [w597 w606 w615 w619 w628] -> w586
              tunnel: w582 -> [w596 w605 w614 w616 w626]
              tunnel: [w596 w605 w614 w618 w627] -> w587
              tunnel: w581 -> [w595 w598 w607 w624 w633]
              tunnel: w580 -> [w594 _ w610 w623 w632]
              tunnel: [w595 w600 w609 w624 w633] -> w585
              tunnel: [w594 w599 w608 w623 w632] -> w584
              tunnel: w579 -> [_ w601 _ _ _]
              frame Default {
              }
              frame "Up" {
                n245 = Subtract(x=w601, y=w598) -> (x-y=w603:dbl)
                n246 = Multiply(x=w603, y=0.05) -> (x*y=w602:dbl)
                n247 = Subtract(x=w602, y=w601) -> (x-y=w599:dbl)
                n248 = Add(x=w598, y=w602) -> (x+y=w600:dbl)
              }
              frame "Down" {
                n249 = Subtract(x=w610, y=w607) -> (x-y=w612:dbl)
                n250 = Multiply(x=w612, y=0.05) -> (x*y=w611:dbl)
                n251 = Add(x=w611, y=w610) -> (x+y=w608:dbl)
                n252 = Subtract(x=w607, y=w611) -> (x-y=w609:dbl)
              }
              frame "Left" {
                n253 = Subtract(x=w616, y=w622) -> (x-y=w620:dbl)
                n254 = Multiply(x=w620, y=0.05) -> (x*y=w617:dbl)
                n255 = Subtract(x=w622, y=w617) -> (x-y=w619:dbl)
                n256 = Add(x=w617, y=w616) -> (x+y=w618:dbl)
              }
              frame "Right" {
                n257 = Subtract(x=w626, y=w631) -> (x-y=w629:dbl)
                n258 = Multiply(x=w629, y=0.05) -> (x*y=w625:dbl)
                n259 = Add(x=w631, y=w625) -> (x+y=w628:dbl)
                n260 = Subtract(x=w626, y=w625) -> (x-y=w627:dbl)
              }
            }
            n261 = property on="Waveform Graph" class="WFGraph (strict)"("YScale.Maximum"=w584) -> ()  [unwired: 2 in, 2 out]
            n262 = property on="Waveform Graph" class="WFGraph (strict)"("YScale.Minimum"=w585) -> ()  [unwired: 2 in, 2 out]
            n263 = property on="Waveform Graph" class="WFGraph (strict)"("XScale.Minimum"=w586) -> ()  [unwired: 2 in, 2 out]
            n264 = property on="Waveform Graph" class="WFGraph (strict)"("XScale.Maximum"=w587) -> ()  [unwired: 2 in, 2 out]
          }
          event Key Repeat {
            # "This event structure allows user to zoom in and out using the arrow keys. Key down and key repeat have the same functions so that the user can either zoom once or hold the arrow down to zoom rapidly."
            n265 = event-data() -> ("VKey"=w645:T8)  [unwired: 1 in]
            n266 = property on="Waveform Graph" class="WFGraph (strict)"() -> ("YScale.Maximum"=w646:dbl)  [unwired: 2 in, 2 out]
            n267 = property on="Waveform Graph" class="WFGraph (strict)"() -> ("XScale.Maximum"=w648:dbl)  [unwired: 2 in, 2 out]
            n268 = property on="Waveform Graph" class="WFGraph (strict)"() -> ("YScale.Minimum"=w647:dbl)  [unwired: 2 in, 2 out]
            n269 = property on="Waveform Graph" class="WFGraph (strict)"() -> ("XScale.Minimum"=w649:dbl)  [unwired: 2 in, 2 out]
            n270 = case shown="\"Left\"" w645 {
              tunnel: w649 -> [w659 w668 w677 w684 w693]
              tunnel: [w659 w668 w677 w681 w690] -> w652
              tunnel: w648 -> [w658 w667 w676 w678 w688]
              tunnel: [w658 w667 w676 w680 w689] -> w653
              tunnel: w647 -> [w657 w660 w669 w686 w695]
              tunnel: w646 -> [w656 _ w672 w685 w694]
              tunnel: [w657 w662 w671 w686 w695] -> w651
              tunnel: [w656 w661 w670 w685 w694] -> w650
              tunnel: w644 -> [_ w663 _ _ _]
              frame Default {
              }
              frame "Up" {
                n271 = Subtract(x=w663, y=w660) -> (x-y=w665:dbl)
                n272 = Multiply(x=w665, y=0.05) -> (x*y=w664:dbl)
                n273 = Subtract(x=w664, y=w663) -> (x-y=w661:dbl)
                n274 = Add(x=w660, y=w664) -> (x+y=w662:dbl)
              }
              frame "Down" {
                n275 = Subtract(x=w672, y=w669) -> (x-y=w674:dbl)
                n276 = Multiply(x=w674, y=0.05) -> (x*y=w673:dbl)
                n277 = Add(x=w673, y=w672) -> (x+y=w670:dbl)
                n278 = Subtract(x=w669, y=w673) -> (x-y=w671:dbl)
              }
              frame "Left" {
                n279 = Subtract(x=w678, y=w684) -> (x-y=w682:dbl)
                n280 = Multiply(x=w682, y=0.05) -> (x*y=w679:dbl)
                n281 = Subtract(x=w684, y=w679) -> (x-y=w681:dbl)
                n282 = Add(x=w679, y=w678) -> (x+y=w680:dbl)
              }
              frame "Right" {
                n283 = Subtract(x=w688, y=w693) -> (x-y=w691:dbl)
                n284 = Multiply(x=w691, y=0.05) -> (x*y=w687:dbl)
                n285 = Add(x=w693, y=w687) -> (x+y=w690:dbl)
                n286 = Subtract(x=w688, y=w687) -> (x-y=w689:dbl)
              }
            }
            n287 = property on="Waveform Graph" class="WFGraph (strict)"("YScale.Maximum"=w650) -> ()  [unwired: 2 in, 2 out]
            n288 = property on="Waveform Graph" class="WFGraph (strict)"("YScale.Minimum"=w651) -> ()  [unwired: 2 in, 2 out]
            n289 = property on="Waveform Graph" class="WFGraph (strict)"("XScale.Minimum"=w652) -> ()  [unwired: 2 in, 2 out]
            n290 = property on="Waveform Graph" class="WFGraph (strict)"("XScale.Maximum"=w653) -> ()  [unwired: 2 in, 2 out]
          }
          event "Discard&Continue": Value Change {
            # "Forget about the current wave and collect a new one."
            n291 = event-data() -> ("NewVal"=w698:bool)  [unwired: 1 in, 4 out]
          }
          event "StartOver": Value Change {
            w704 = T9 []  # DescribeWave
            # "Deletes the waveform specified by the path field."
            n292 = event-data() -> ("NewVal"=w701:bool)  [unwired: 1 in, 4 out]
            n293 = call <vilib>:"Check if File or Folder Exists.vi"("path"=w705) -> ("error out"=w707:errorcluster, "file or folder exists?"=w706:bool, "dup path"=w708:path)  [unwired: 8 in]
            n294 = case shown="False" w706 {
              selector: w706 -> [_ w711]
              tunnel: w708 -> [_ w714]
              tunnel: w707 -> [_ w713]
              frame False {
                n295 = One Button Dialog(message="File does not exist and cannot be deleted.", button name ("OK")="OK") -> ()  [unwired: 1 out]
              }
              frame True {
                n296 = Delete(path (use dialog)=w714, confirm (F)=w711, error in=w713) -> (error out=w712:errorcluster)  [unwired: 2 in, 2 out]
                n297 = call <vilib>:"Simple Error Handler.vi"("error in (no error)"=w712) -> ()  [unwired: 4 in, 5 out]
              }
            }
          }
        }
        n298 = Build Array(w502, w501, w500, w499) -> (w498:bool[])
        n299 = Bundle By Name(cluster=w535, "DescribeWave"=w504) -> (w534:T1)
        n300 = Select(t=w492, s=w491, f=w493) -> (s? t:f=w494:T2)
        "Time" <- w523
        "Date" <- w524
      }
      frame "write to file" {
        # "2=Save&Finish\n3=Save&Continue"
        n301 = Unbundle By Name(w748) -> ("data"=w736:dbl[][], "LastGrabbedSrate"=w737:dbl, "DescribeWave"=w747:T9)  [unwired: 6 out]
        n302 = Index Array(array=w747) -> (element=w734:T10)  [unwired: 1 in]
        n303 = Unbundle By Name(w734) -> ("Polarity 2"=w720:bool)
        n304 = Index Array(array=w736) -> (element=w722:dbl[])  [unwired: 2 in]
        n305 = call "Polarize.vi"("Polarity"=w720, "Wave array"=w722) -> ("Inverse Wave Array"=w723:dbl[])  [unwired: 9 in]
        n306 = Boolean To (0,1)(Boolean=w720) -> (0, 1=w733:i16)
        n307 = Unbundle By Name(w734) -> ("Time 2"=w746:string, "Date 2"=w745:string, "Specimen 2"=w744:string, "Location 2"=w743:string, "Species 2"=w742:string, "Temp 2"=w741:string, "Gain 2"=w724:dbl, "Coupling 2"=w740:bool, "Comments 2"=w739:string)
        n308 = Array To Cluster(array=w725) -> (cluster=w727:T11)
        n309 = Multiply(x=w724, y=w723) -> (x*y=w735:dbl[])
        n310 = To Byte Integer(number=w733) -> (8bit integer=w732:i8)
        n311 = Unbundle By Name(w727) -> ("[2]"=w719:bool, "[3]"=w726:bool)
        n312 = Build Array(w735) -> (w721:dbl[][])
        n313 = property on="Timed" class="Bool (strict)"() -> ("Value"=w715:bool)  [unwired: 2 in, 2 out]
        n314 = Bundle("Time 2"=w746, "Date 2"=w745, "Specimen 2"=w744, "Location 2"=w743, "Species 2"=w742, "Temp 2"=w741, "Gain 2"=w724, "Coupling 2"=w740, "Comments 2"=w739) -> (w738:T12)  [unwired: 1 in]
        n315 = call "writefile.vi"("Path"=w731, "Save&Continue"=w726, "Save&Finish"=w719, "Polarity"=w732, "Sample Rate"=w737, "Array"=w721, "DescribeWave"=w738) -> ("Path Out"=w730:path, "Enum"=w717:T2)  [unwired: 3 in]
        n316 = case shown="False" w715 {
          tunnel: [w749 w751] -> w718
          tunnel: w717 -> [w749 _]
          tunnel: w716 -> [_ w750]
          frame False {
          }
          frame True {
            n317 = flat-sequence {
              tunnel: w750 -> [w760]
              tunnel: [w755] -> w752
              tunnel: [w768] -> w751
              tunnel: w752 -> [w767]
              frame #0 {
                n318 = property on="Waveforms\nCollected" class="DigNum (strict)"() -> ("Value"=w754:dbl)  [unwired: 2 in, 2 out]
                n319 = Increment(x=w754) -> (x+1=→"Waveforms\nCollected":dbl)
              }
              frame #1 {
                n320 = property on="Number of \nWaveforms" class="DigNum (strict)"() -> ("Value"=w756:dbl)  [unwired: 2 in, 2 out]
                n321 = property on="Waveforms\nCollected" class="DigNum (strict)"() -> ("Value"=w757:dbl)  [unwired: 2 in, 2 out]
                n322 = Equal?(x=w757, y=w756) -> (x = y?=w758:bool)
                n323 = case shown="False" w758 {
                  selector: w758 -> [w761 w765]
                  tunnel: w760 -> [w764 _]
                  tunnel: [w763 0] -> w759
                  tunnel: [w761 w765] -> w755
                  frame False {
                    n324 = Multiply(x=w764, y=1000.0) -> (x*y=w763:dbl)
                  }
                  frame True {
                  }
                }
                n325 = Wait (ms)(milliseconds to wait=w759) -> ()  [unwired: 1 out]
              }
              frame #2 {
                n326 = case shown="True" w767 {
                  tunnel: [eodrecorderstates."capture data" ("Enum") eodrecorderstates."stop" ("Enum")] -> w768
                  frame False {
                  }
                  frame True {
                    w770 = 0.0 ("Value (Signaling)")
                    n327 = property on="Timed" class="Bool (strict)"("Val(Sgnl)"=FALSE ("Value (Signaling)")) -> ()  [unwired: 2 in, 2 out]
                    n328 = property on="Number of \nWaveforms" class="DigNum (strict)"("Val(Sgnl)"=w770) -> ()  [unwired: 2 in, 2 out]
                    n329 = property on="Waveforms\nCollected" class="DigNum (strict)"("Val(Sgnl)"=w770) -> ()  [unwired: 2 in, 2 out]
                  }
                }
              }
            }
          }
        }
        n330 = property on="Path" class="Path"("Val(Sgnl)"=w730) -> ()  [unwired: 2 in, 2 out]
      }
    }
    "Waveform Graph" <- w24
    "Tab Control" <- w41
    n331 = feedback-in #1(w16) -> ()
    n332 = feedback-in #2(w14) -> ()
    n333 = feedback-in #3(w10) -> ()
    n334 = Index Array(array=string[] ["Live Data", "Edit Data", "Previously Acquired Data"], index=w41) -> (element=→"String":string)
    n335 = property on="String" class="Str"("Text.BGColor"=w40) -> ()  [unwired: 2 in, 2 out]
  }
  n336 = property on="Waveform Graph" class="WFGraph (strict)"("XScale.Multiplier"=w1) -> ()  [unwired: 2 in, 2 out]
